vi "Periodic Tasks.vi"(8 "error in":errorcluster) -> ()   [LabVIEW 2020]
doc: "This VI runs in parallel to other tasks. It can contain as many user-defined periodic loops as you need. These can carry out PID or other sorts of timed response."
uses:
  myStates.ctl
  Test VIs/SlipControlStates.ctl
  <vilib>/Rock Robotics/WPI/DriverStation/WPI_DriverStationRobotMode2.ctl
  <vilib>/Rock Robotics/WPI/ThirdParty/REV Robotics/REVLib/Typedef/Spark MAX Control Type.ctl
  4913f956-5bda-4107-8571-b517f3ac16c4.vi
  <vilib>/Rock Robotics/WPI/Utilities/WPI_GetSetVariantRefNum.vi
  <vilib>/Rock Robotics/Network Tables/NT Write Number.vi
  <vilib>/Rock Robotics/Network Tables/NT Read Boolean Array.vi
  <vilib>/Rock Robotics/Network Tables/NT Read Number.vi
  <vilib>/Rock Robotics/Network Tables/NT Read Boolean.vi
  Robot Global Data.vi
  <vilib>/Rock Robotics/Network Tables/NT Write Numeric Array.vi
  <vilib>/Rock Robotics/Network Tables/NT Write String.vi
  <vilib>/Rock Robotics/Network Tables/NT Write Boolean Array.vi
  <vilib>/Comparison/Equal/Equal Functor/Equal Functor.lvclass
panel:
  out "Drivetrain Currents":dbl[](array[numeric])
  out "DEP Right Running Ave":dbl
  out "DEP Left Running Ave":dbl
  out "EXC Right Running Ave":dbl
  out "EXC Left Running Ave":dbl
  # "Click here to set max"
  # "Click here to set min"
  # "Click here to set max"
  # "Click here to set min"
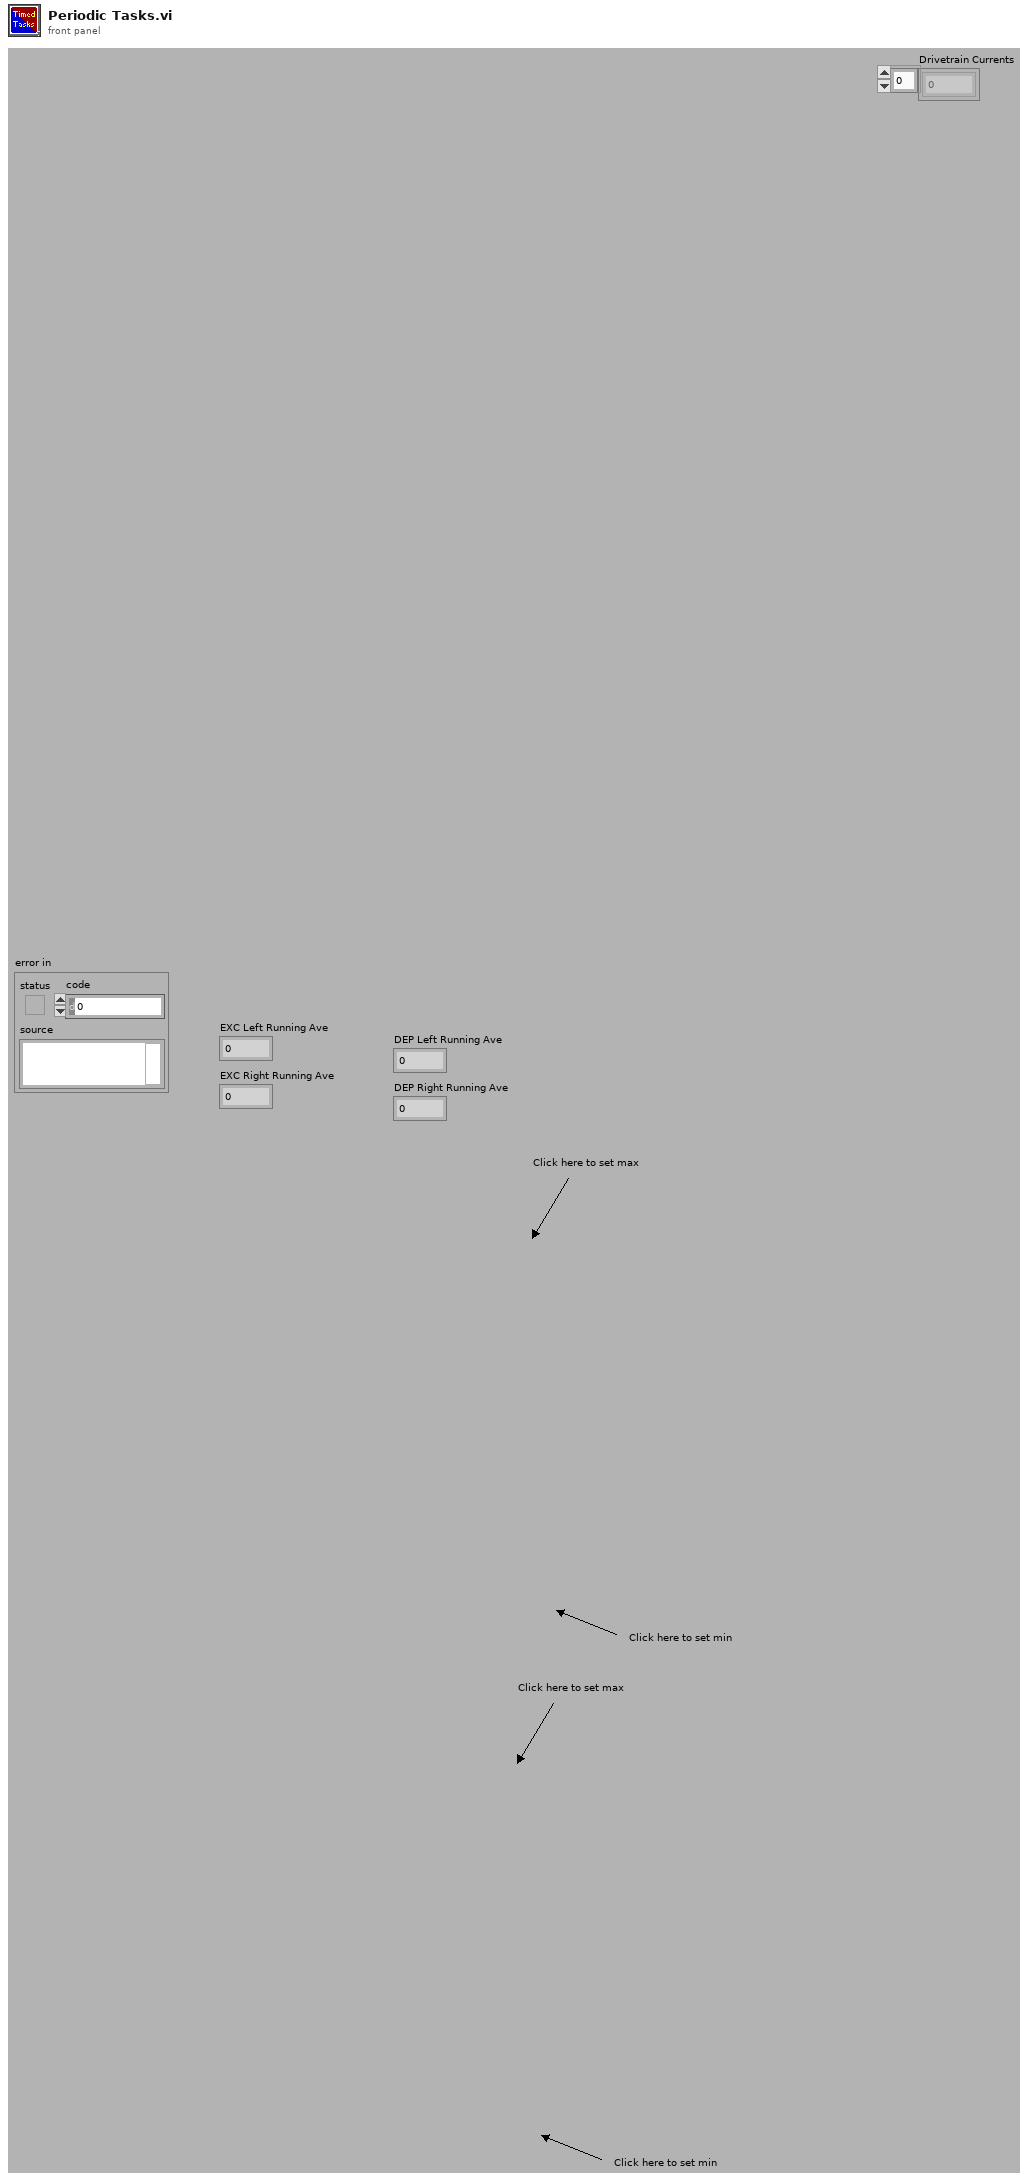
[diagram p1: front panel]
types:
  T1 = typedef "SlipControlStates.ctl" = enum16{"Init", "Grab Time", "Wait", "Grab Time (good)", "Waiting (while run)", "Check", "Grab Time (bad)", "Wait (No Run)"}
  T2 = typedef "myStates.ctl" = enum16{"Init", "Manual Control", "Autonomous Traversal", "Avoid Left", "Avoid Right", "Return to Trench", "EXC Deploy", "EXC Excavate", "EXC Inch", "EXC Index", "EXC Retract", "Drive to Dep", "Approach Berm", "HAD Deploy", "HAD Deposit", "HAD Retract", "Return to EXC"}
  T3 = typedef "WPI_AnalogChannelDevRef.ctl" = cluster{"DevStatus":errorcluster, "Analog Channel":T4}
  T4 = typedef "FPGA_AIChannel.ctl" = enum8{"AI 0", "AI 1", "AI 2", "AI 3", "AI MXP 0", "AI MXP 1", "AI MXP 2", "AI MXP 3", "Invalid"}
  T5 = typedef "WPI_JoystickDevRef.ctl" = cluster{"Device":T6}
  T6 = typedef "WPI_JoystickDeviceEnum.ctl" = enum16{"USB 0", "USB 1", "USB 2", "USB 3", "USB 4", "USB 5"}
  T7 = typedef "Spark MAX Control Type.ctl" = enum16{"Percent VBus", "Voltage", "Velocity", "Position", "Smart Motion", "Current", "Smart Velocity"}
  T8 = typedef "WPI_DriverStationRobotMode2.ctl" = enum16{"Autonomous Disabled", "Autonomous Enabled", "Teleop Disabled", "Teleop Enabled", "Disconnected", "Finish", "Test Disabled", "Test Enabled", "Emergency Stopped"}
  T9 = cluster{"Buttons[0]":bool, "Buttons[1]":bool, "Buttons[2]":bool, "Buttons[3]":bool, "Buttons[4]":bool, "Buttons[5]":bool, "Buttons[6]":bool, "Buttons[7]":bool, "Buttons[8]":bool}
  T10 = cluster{"Axes[0]":dbl, "Axes[1]":dbl, "Axes[2]":dbl, "Axes[3]":dbl, "Axes[4]":dbl, "Axes[5]":dbl, "Axes[6]":dbl, "Axes[7]":dbl, "Axes[8]":dbl}
  T11 = cluster{"Yaw":dbl, "Roll":dbl, "Pitch":dbl, "Heading":dbl, "Fused Heading":dbl}
  T12 = cluster{"Velocity X":dbl, "Velocity Y":dbl, "Velocity Z":dbl, "Displacement X":dbl, "Displacement Y":dbl, "Displacement Z":dbl}
  T13 = typedef "Z900_navX_Flags_HardwareRevTypeDef.ctl" = u8
  T14 = typedef "Z900_navX_Flags_OmnimountConfigTypeDef.ctl" = u8
  T15 = cluster{"Board":cluster{"Who Am I":u8, "Hardware Revision":T13, "Firmware Major Version":u8, "Firmware Minor Version":u8}, "Capability":cluster{"OMNIMOUNT":bool, "YAW_RESET":bool, "VEL_AND_DISP":bool}, "Omnimount Config":T14}
  T16 = cluster{bool[], dbl, dbl, "Left axis value":dbl, "Right axis value":dbl, dbl, "Enum":T1, "current (A)":dbl, "current (A)":dbl, "current (A)":dbl, "current (A)":dbl}
  T17 = cluster{"Want to Drive Out":bool[], "Time Out":dbl, "Front Left Speed Out":dbl, "Back Left Speed Out":dbl, "Front Right Speed Out":dbl, "Back Right Speed Out":dbl, "State Out":T1}
  T18 = typedef "WPI_MotorControlDeviceRef.ctl" = cluster{"DeviceStatus":errorcluster, "Type":T19, "PWM":cluster{"PWM Channel":T20, "DeadBand":T21}, "CAN":cluster{"Device Number":u8, "SetOutput VI Ref":variant, "GetOutput VI Ref":variant, "Enable VI Ref":variant, "Disable VI Ref":variant, "Data":variant}, "Invert":bool, "DIO PWM":cluster{"PWM \"Enable\" Channel":T20, "DIOChannel":T22, "PWM Rate":dbl}}
  T19 = typedef "WPI_MotorControlType.ctl" = enum16{"PWM", "CAN", "DIO PWM"}
  T20 = typedef "FPGA_DIOPWMChannel.ctl" = enum8{"PWM 0", "PWM 1", "PWM 2", "PWM 3", "PWM 4", "PWM 5", "PWM 6", "PWM 7", "PWM 8", "PWM 9", "PWM MXP 0", "PWM MXP 1", "PWM MXP 2", "PWM MXP 3", "PWM MXP 4", "PWM MXP 5", "PWM MXP 6", "PWM MXP 7", "PWM MXP 8", "PWM MXP 9", "Invalid"}
  T21 = typedef "WPI_PWMDeadband.ctl" = cluster{"Name":string, "maxPositivePwm":i32, "minPositivePwm":i32, "centerPwm":i32, "maxNegativePwm":i32, "minNegativePwm":i32, "angularRange":u16}
  T22 = typedef "FPGA_DIOChannel.ctl" = enum8{"DIO 0", "DIO 1", "DIO 2", "DIO 3", "DIO 4", "DIO 5", "DIO 6", "DIO 7", "DIO 8", "DIO 9", "DIO MXP 0", "DIO MXP 1", "DIO MXP 2", "DIO MXP 3", "DIO MXP 4", "DIO MXP 5", "DIO MXP 6", "DIO MXP 7", "DIO MXP 8", "DIO MXP 9", "DIO MXP 10", "DIO MXP 11", "DIO MXP 12", "DIO MXP 13", "DIO MXP 14", "DIO MXP 15", "SPI Port CS1", "SPI Port CS2", "SPI Port CS3", "SPI Port MISO", "SPI Port MOSI", "Invalid"}
  T23 = typedef "WPI_DigitalOutputDevRef.ctl" = cluster{"DIO Channel":T22, "DevStatus":errorcluster}
  T24 = typedef "WPI_RobotDriveDevRef.ctl" = cluster{"DevStatus":errorcluster, "Motors[]":T18[], "Square Inputs":bool, "Max Output":dbl}
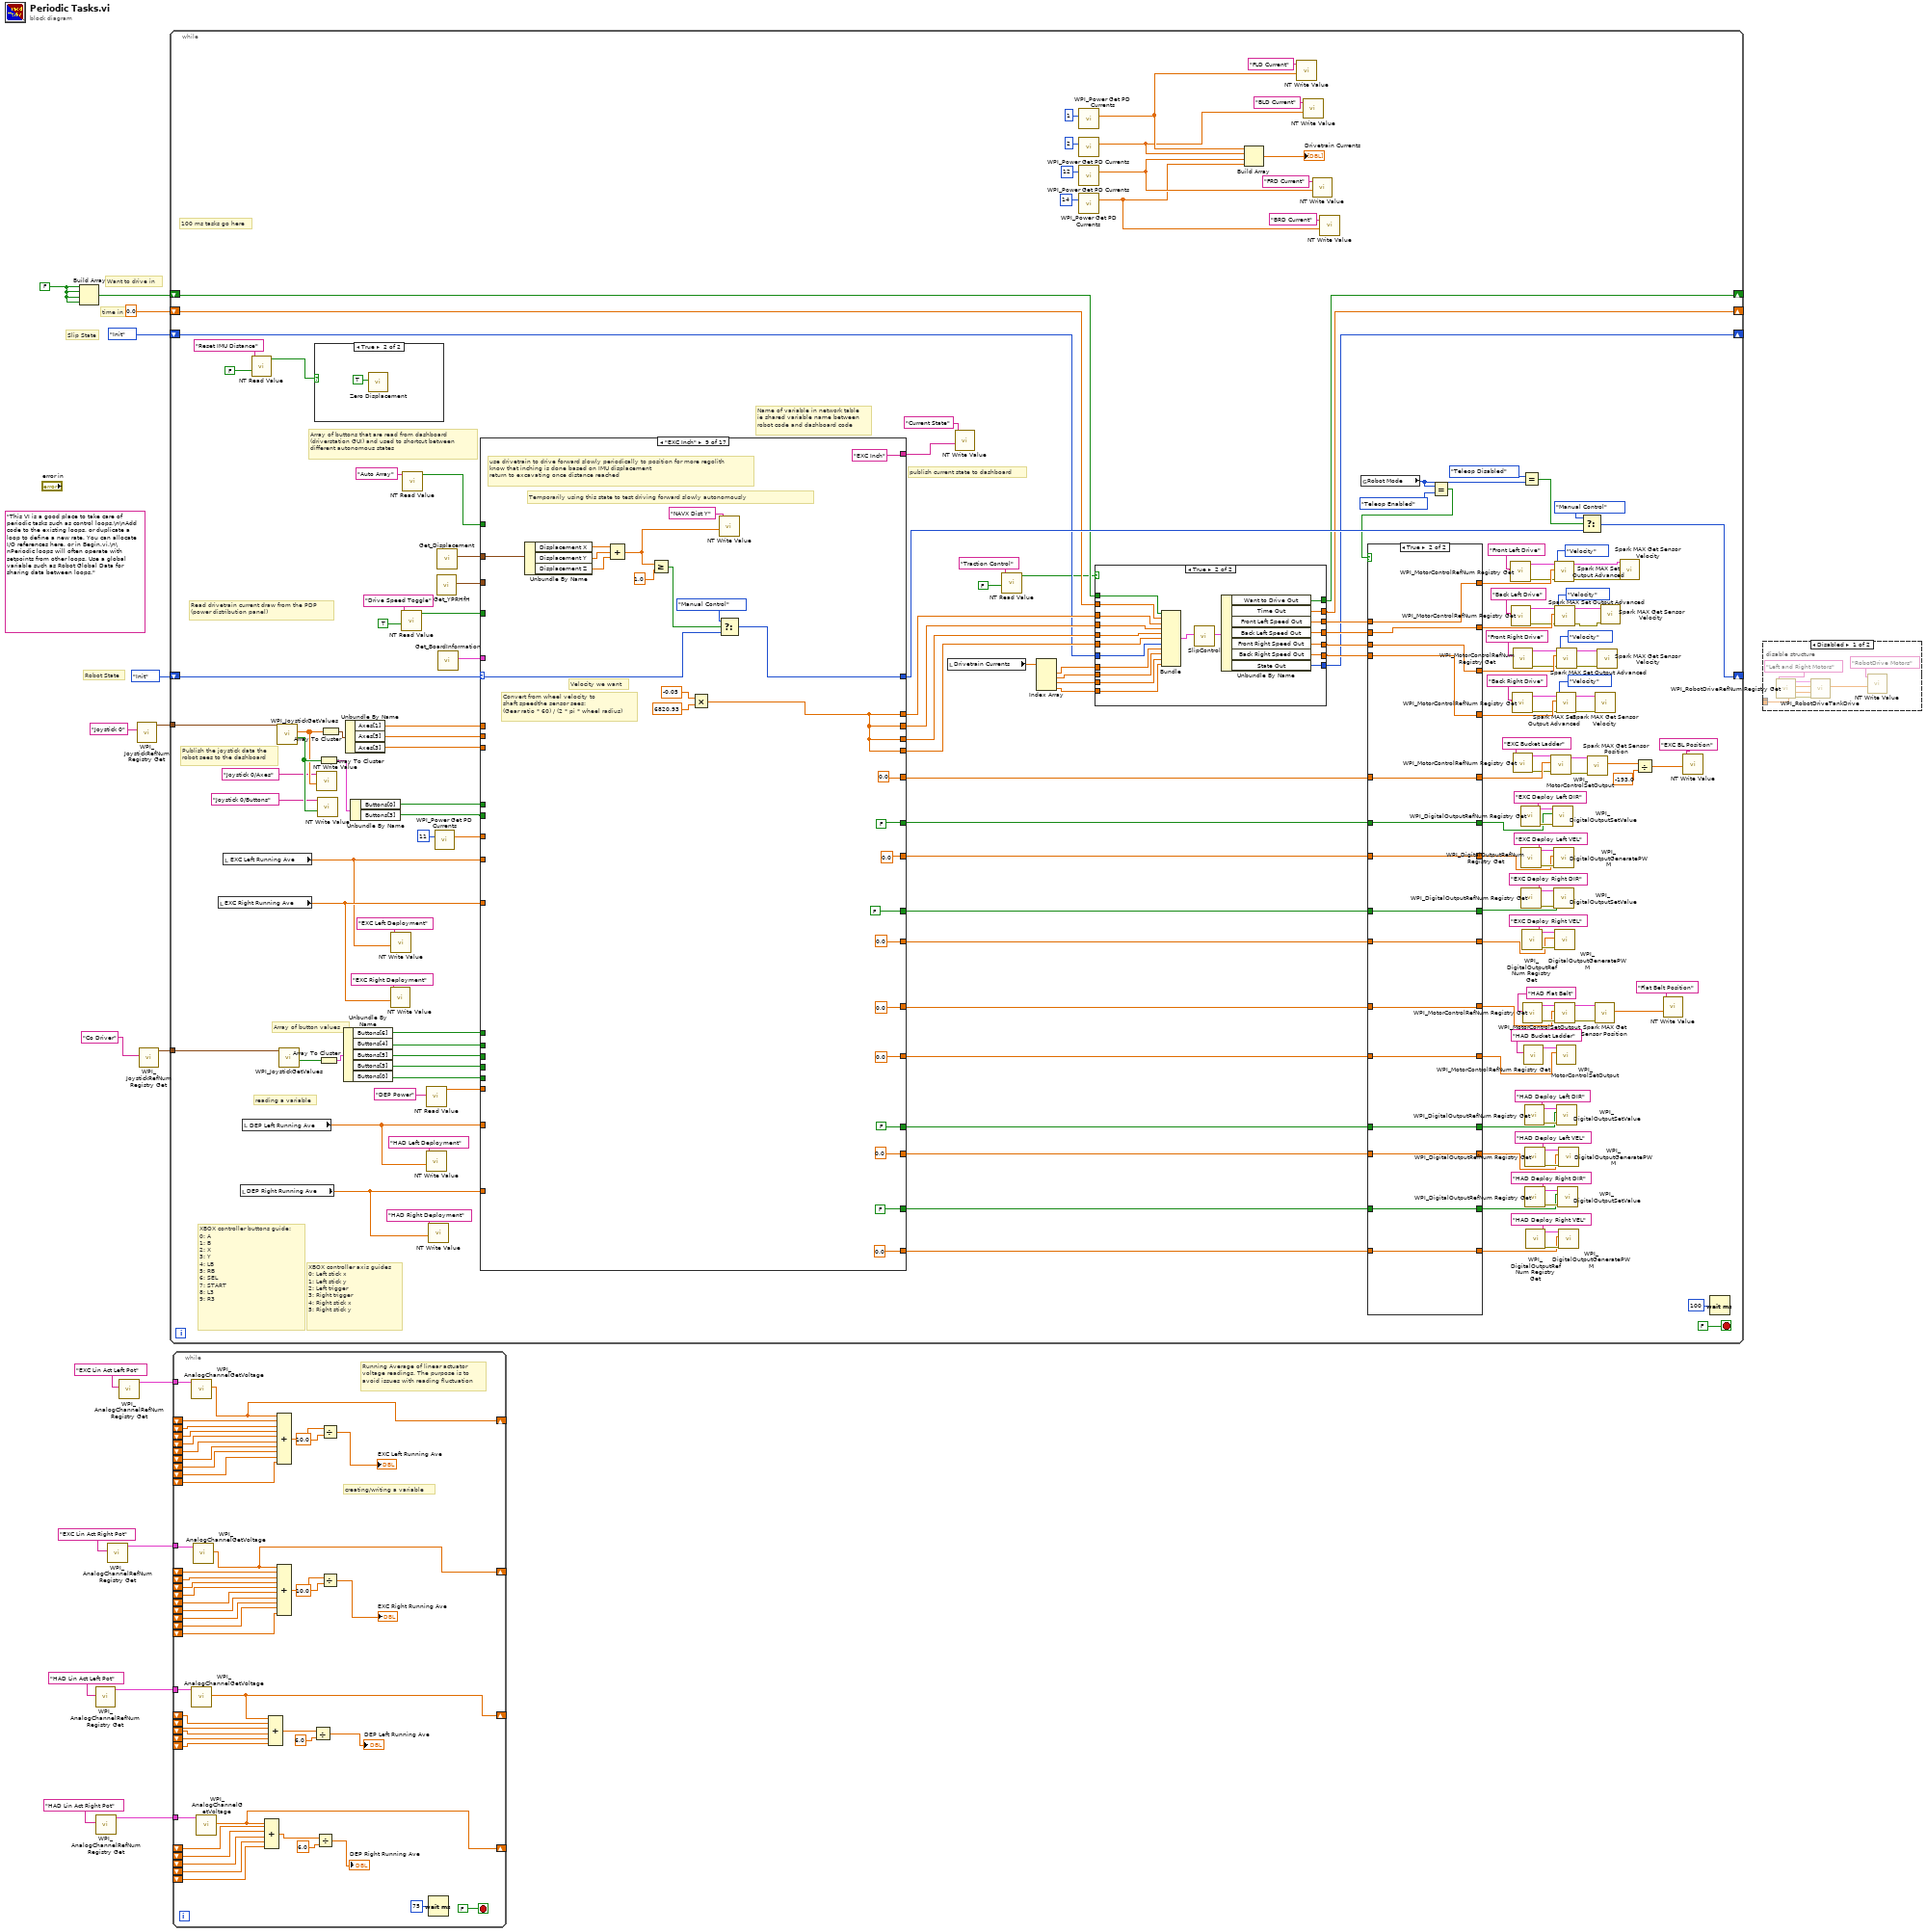
[diagram p0: block diagram]
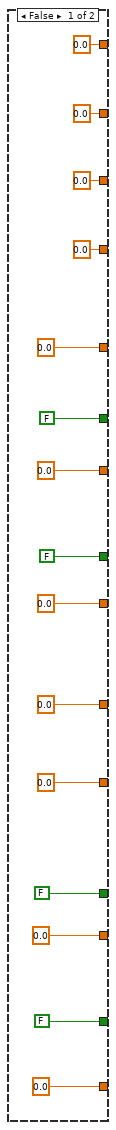
[diagram p5: hidden frame]
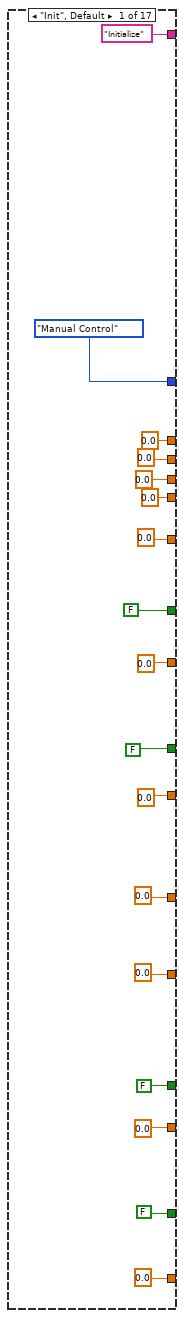
[diagram p6: hidden frame]
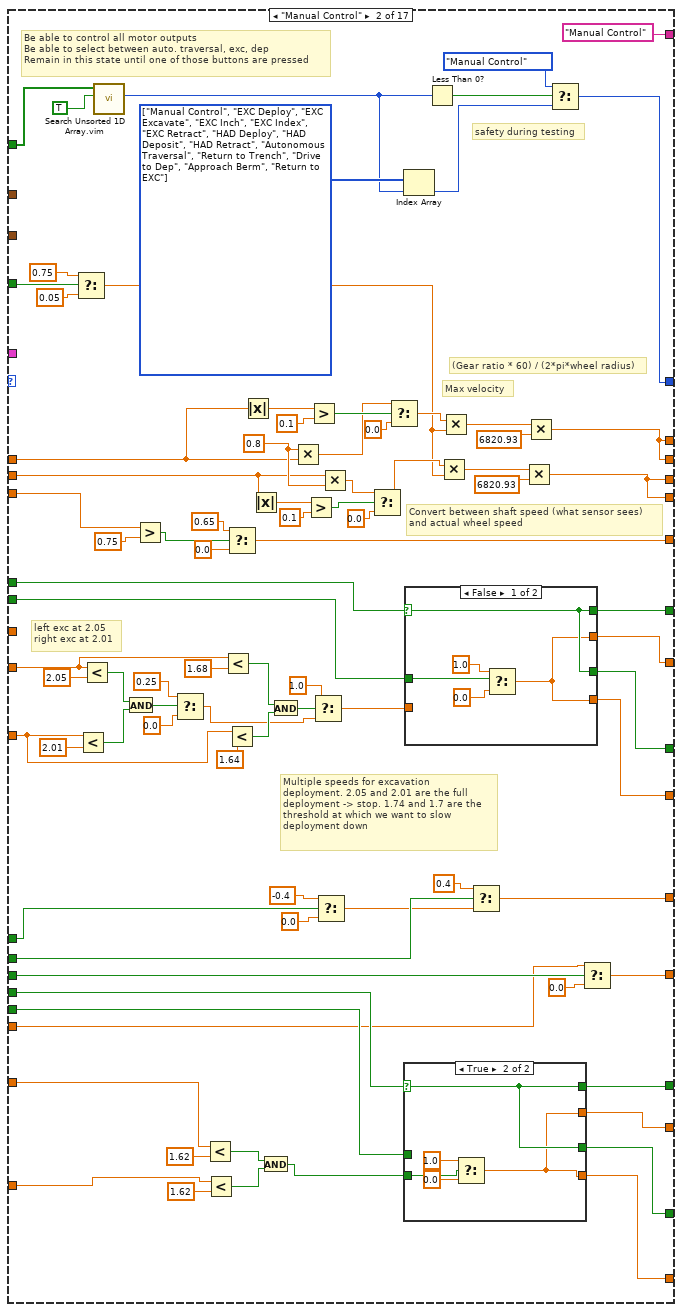
[diagram p7: hidden frame]
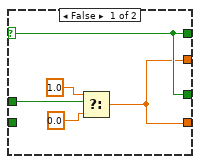
[diagram p8: hidden frame]
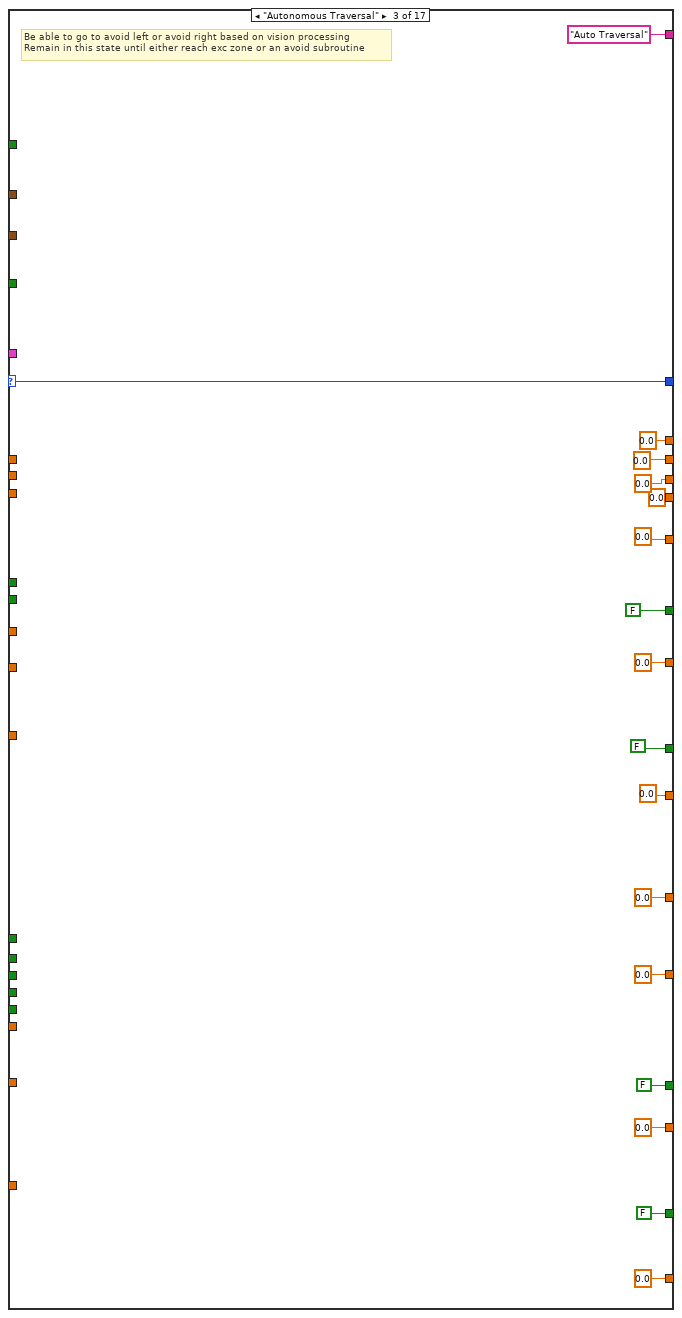
[diagram p10: hidden frame]
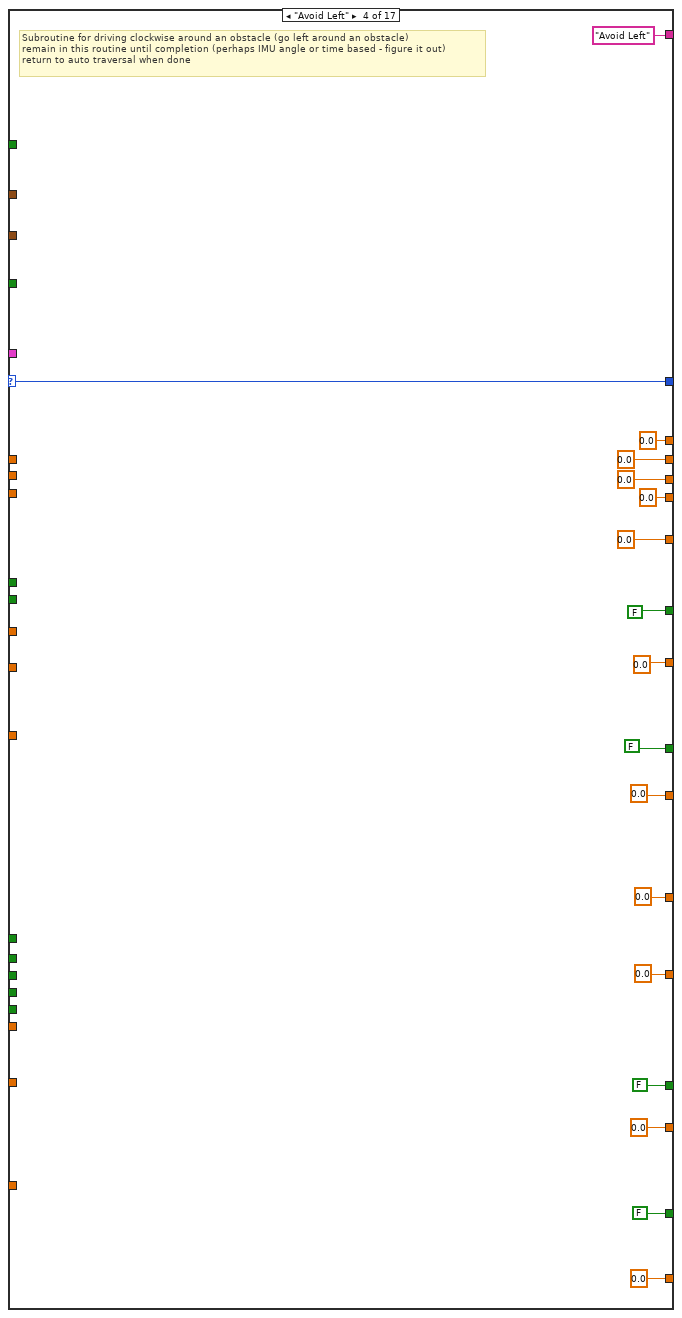
[diagram p11: hidden frame]
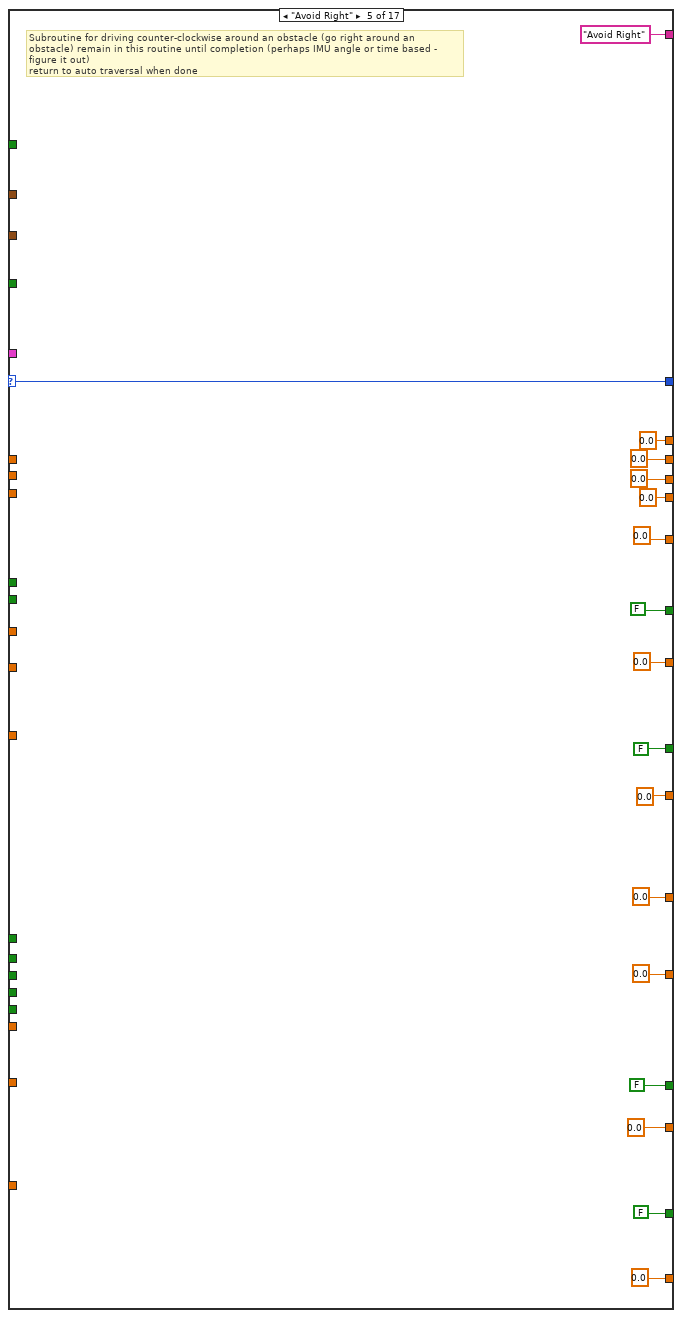
[diagram p12: hidden frame]
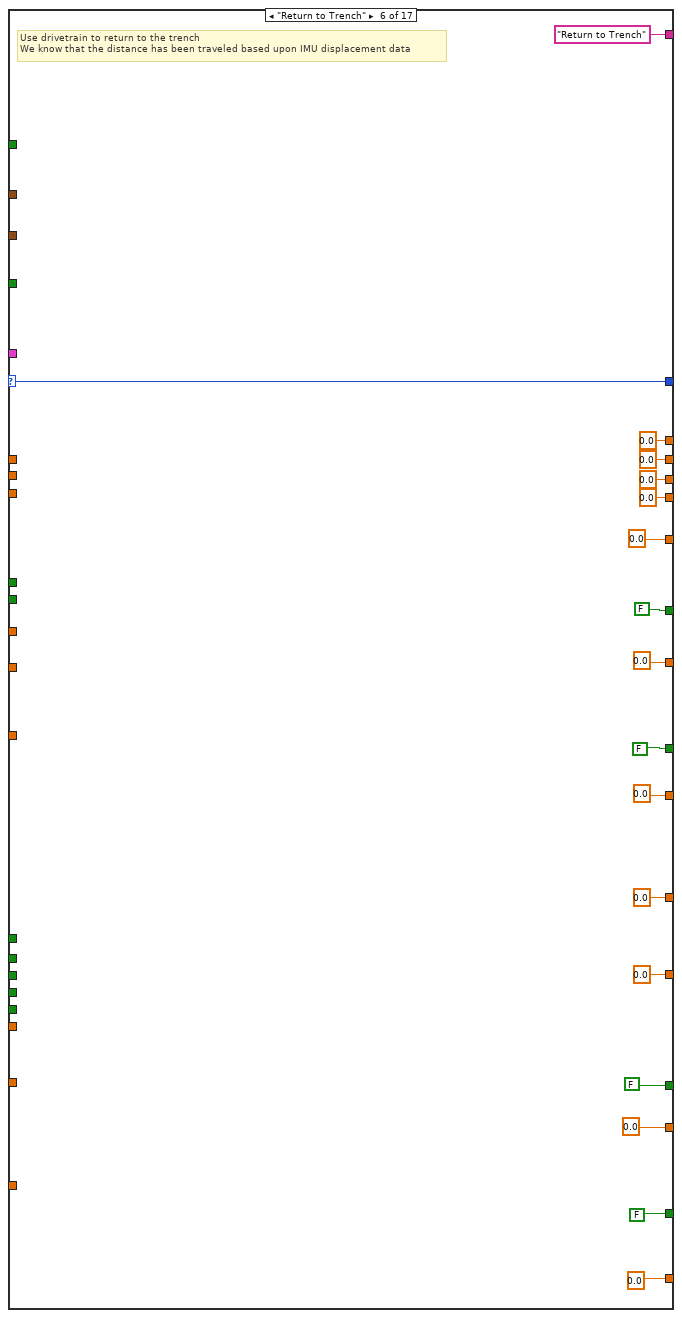
[diagram p13: hidden frame]
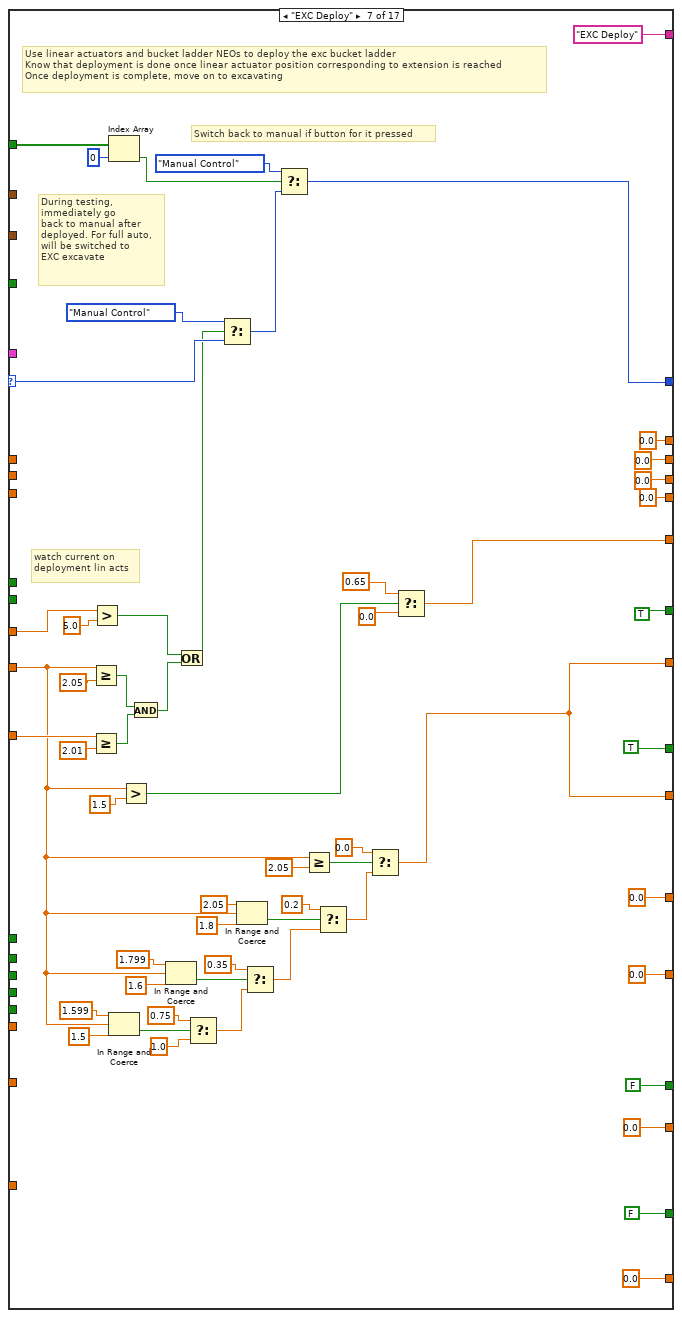
[diagram p14: hidden frame]
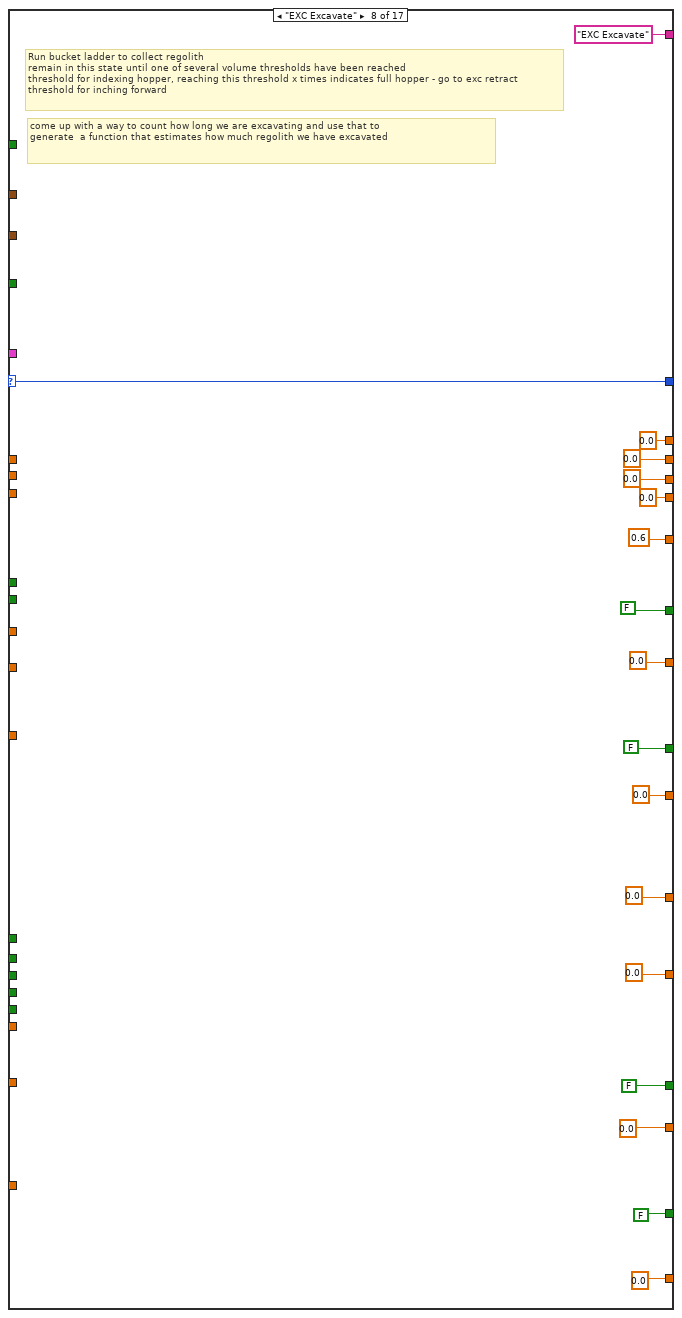
[diagram p15: hidden frame]
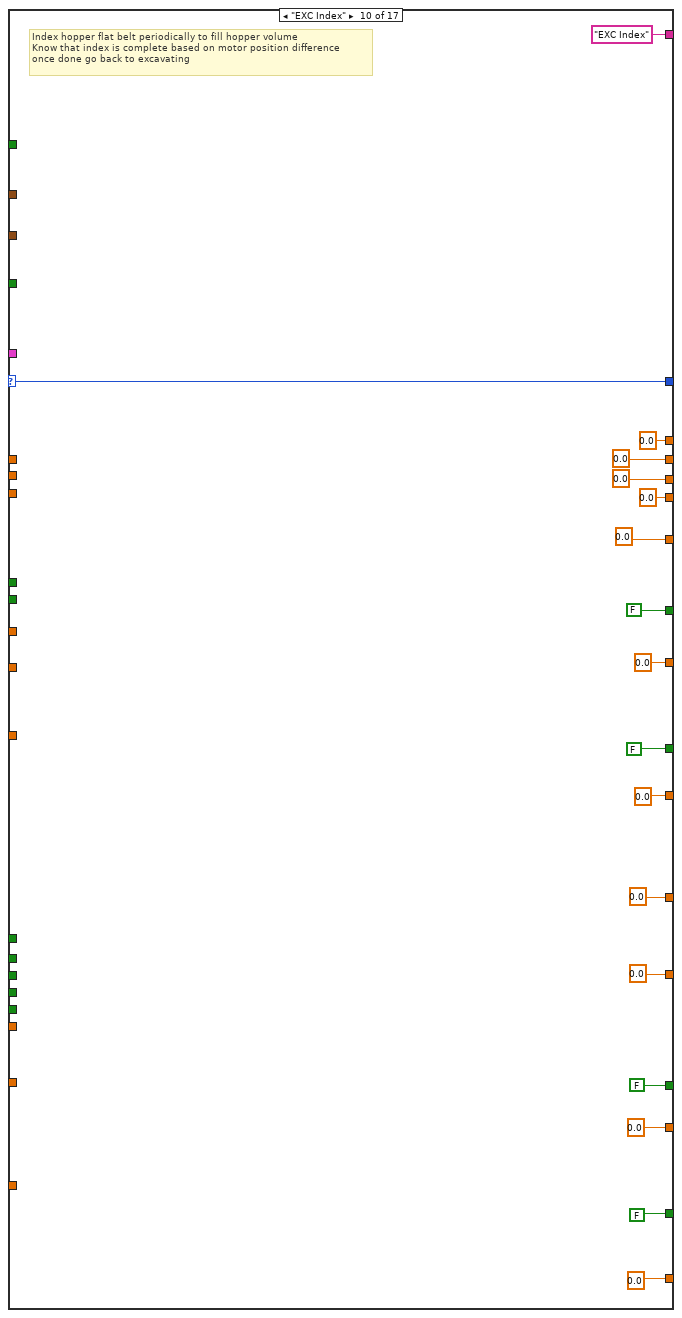
[diagram p16: hidden frame]
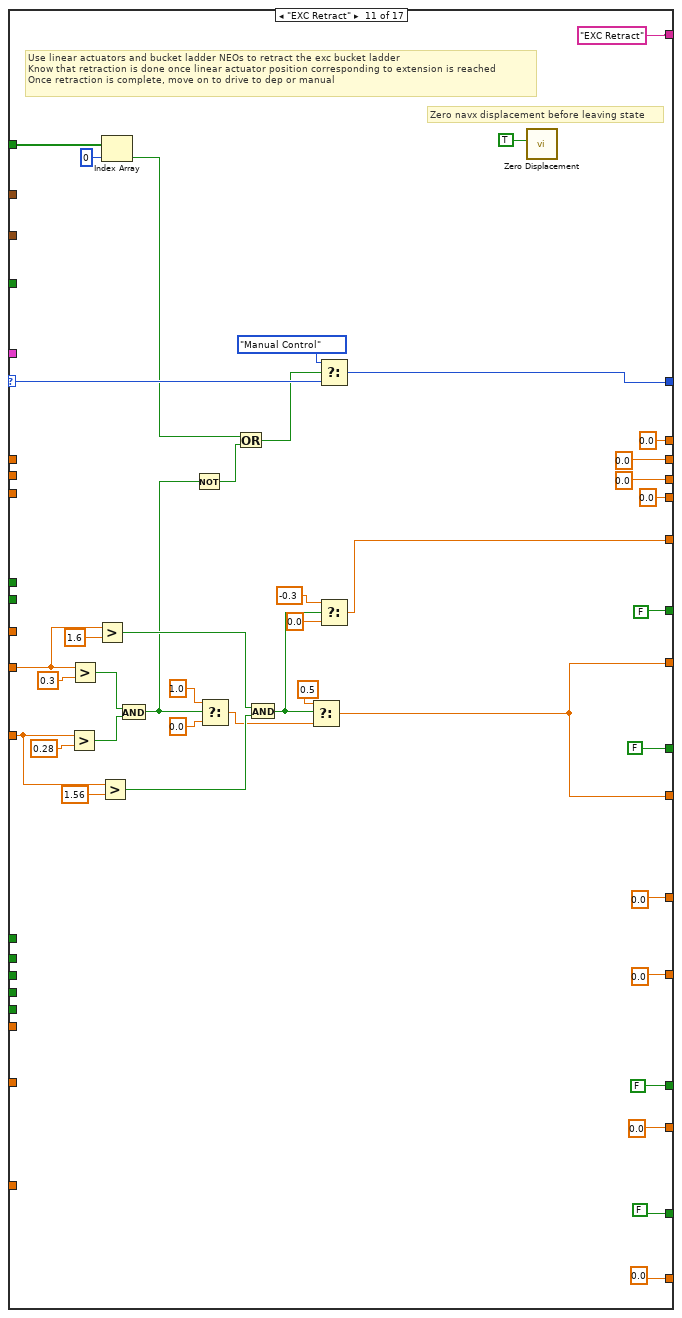
[diagram p17: hidden frame]
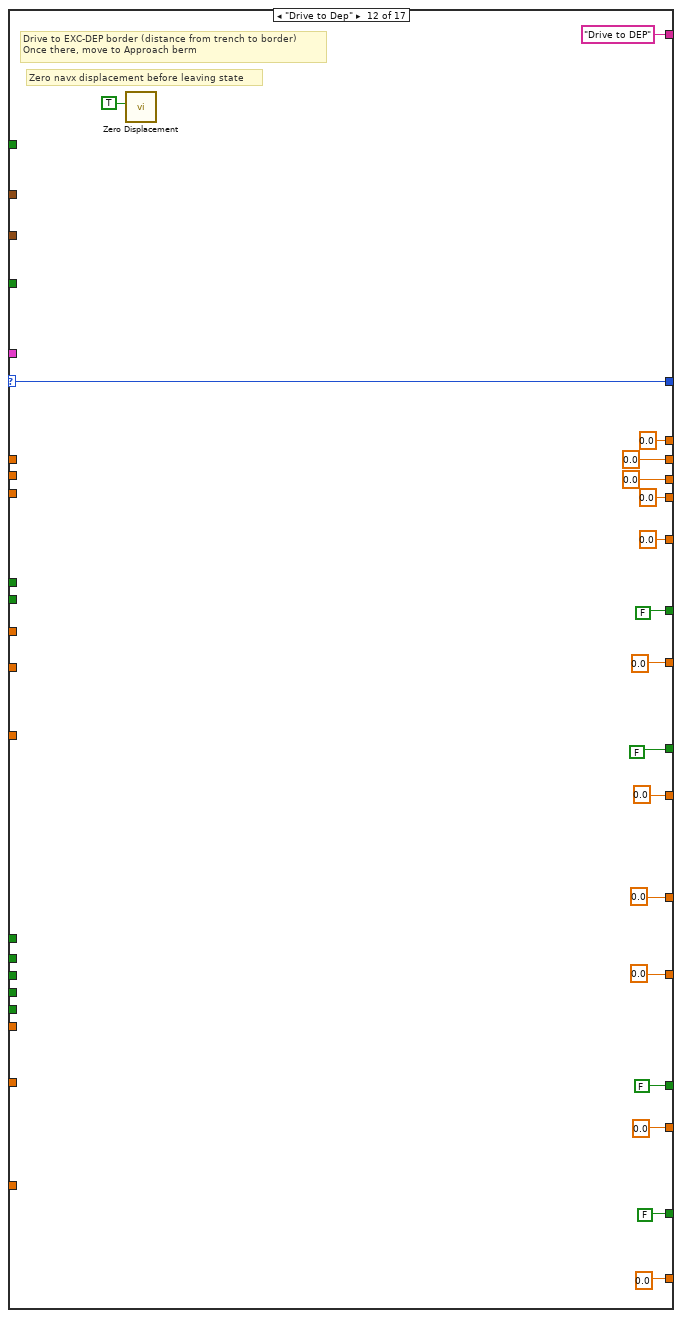
[diagram p18: hidden frame]
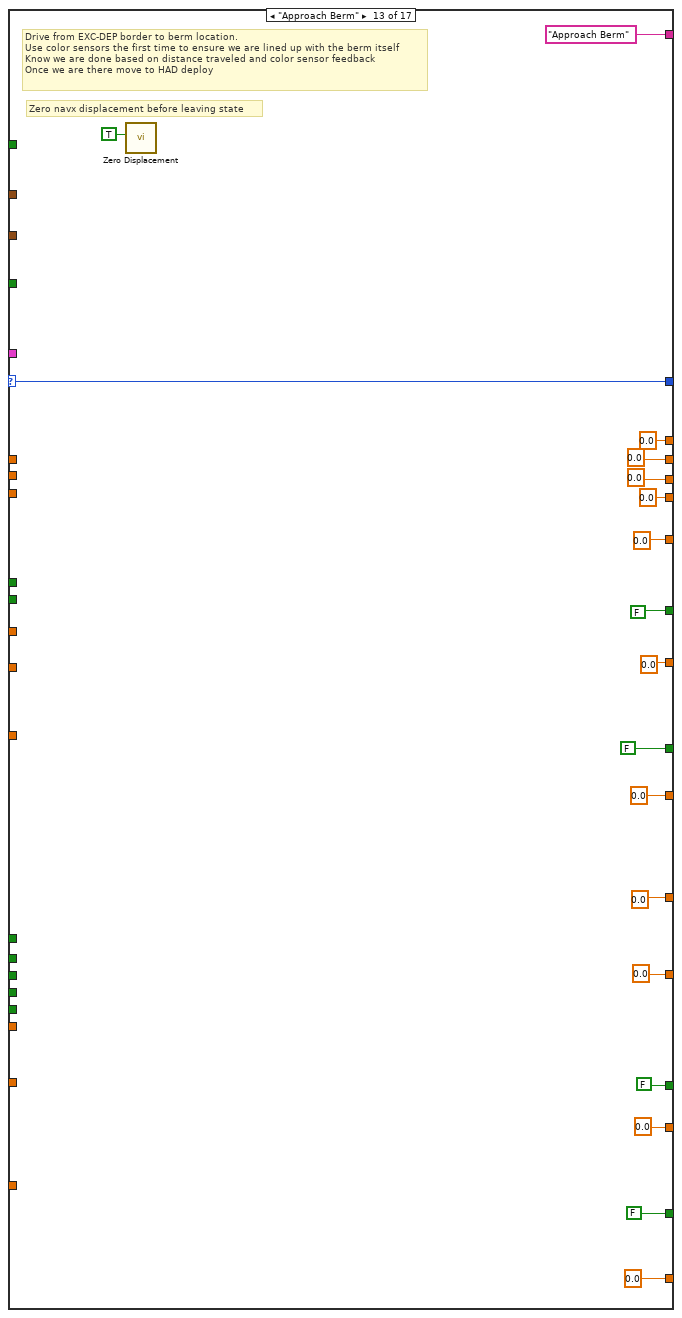
[diagram p19: hidden frame]
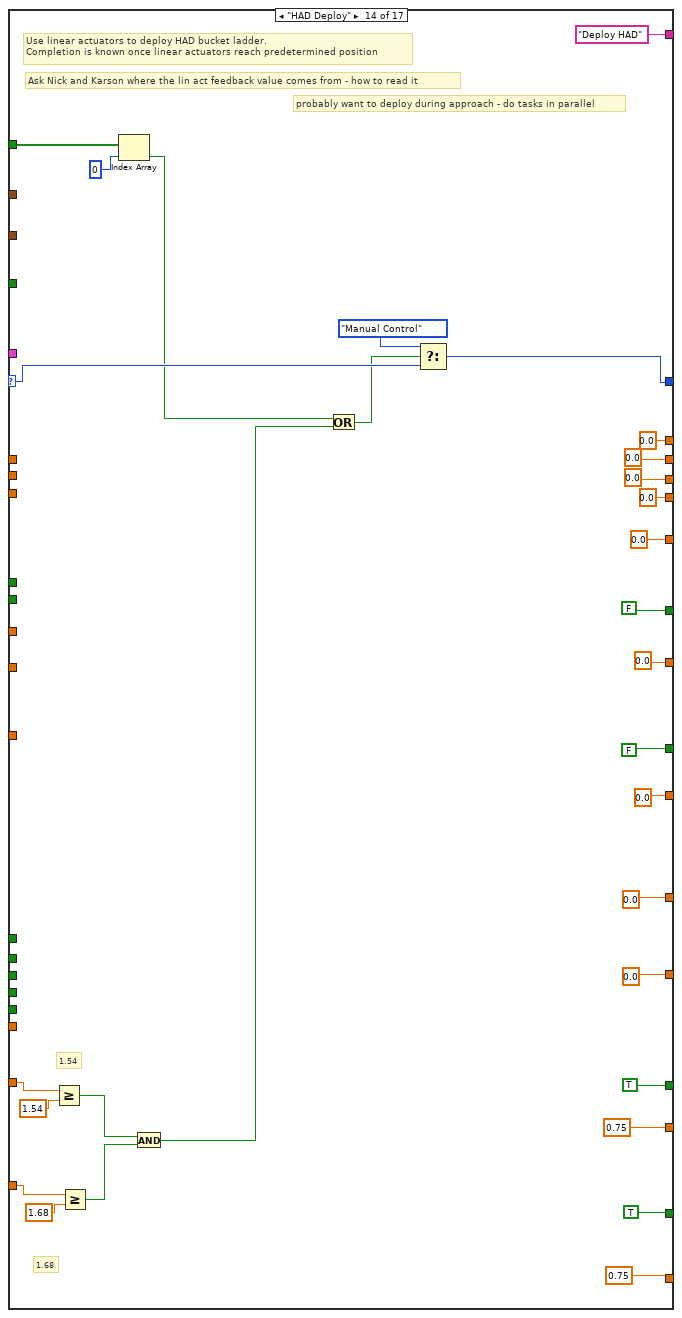
[diagram p20: hidden frame]
diagram:
  w4 = FALSE
  (unwired) "This VI is a good place to take care of periodic tasks such as control loops.\n\nAdd code to the existing loops, or duplicate a loop to define a new rate. You can allocate I/O references here, or in Begin.vi.\n\nPeriodic loops will often operate with setpoints from other loops. Use a global variable such as Robot Global Data for sharing data between loops."
  # "Slip State"
  # "time in"
  # "Want to drive in"
  # "Robot State"
  n1 = Build Array(w4, w4, w4, w4) -> (w3:bool[])
  n2 = call <vilib>:"WPI_AnalogChannelRefNum Registry Get.vi"("refnum name"="HAD Lin Act Left Pot") -> ("AIDeviceRef"=w6:T3)  [unwired: 9 in, 1 out]
  n3 = call <vilib>:"WPI_AnalogChannelRefNum Registry Get.vi"("refnum name"="HAD Lin Act Right Pot") -> ("AIDeviceRef"=w5:T3)  [unwired: 9 in, 1 out]
  n4 = call <vilib>:"WPI_AnalogChannelRefNum Registry Get.vi"("refnum name"="EXC Lin Act Right Pot") -> ("AIDeviceRef"=w7:T3)  [unwired: 9 in, 1 out]
  n5 = call <vilib>:"WPI_AnalogChannelRefNum Registry Get.vi"("refnum name"="EXC Lin Act Left Pot") -> ("AIDeviceRef"=w8:T3)  [unwired: 9 in, 1 out]
  n6 = call <vilib>:"WPI_JoystickRefNum Registry Get.vi"("refnum name"="Joystick 0") -> ("JoystickDevRef"=w15:T5)  [unwired: 1 in, 9 out]
  n7 = call <vilib>:"WPI_JoystickRefNum Registry Get.vi"("refnum name"="Co Driver") -> ("JoystickDevRef"=w13:T5)  [unwired: 1 in, 9 out]
  n8 = while {
    shift-right: [w105] -> _
    shift-left: myStates."Init" -> [w110]
    tunnel: w15 -> [w152]
    tunnel: w13 -> [w151]
    shift-right: [w40] -> _
    shift-left: w3 -> [w59]
    shift-right: [w39] -> _
    shift-left: 0.0 -> [w58]
    shift-right: [w38] -> _
    shift-left: SlipControlStates."Init" ("Enum") -> [w53]
    stop <- FALSE stop-if-true
    # "Read drivetrain current draw from the PDP\n(power distribution panel)"
    # "reading a variable"
    # "Name of variable in network table\nie shared variable name between\nrobot code and dashboard code"
    # "publish current state to dashboard"
    # "XBOX controller axis guides\n0: Left stick x\n1: Left stick y\n2: Left trigger\n3: Right trigger\n4: Right stick x\n5: Right stick y"
    # "XBOX controller buttons guide:\n0: A\n1: B\n2: X\n3: Y\n4: LB\n5: RB\n6: SEL\n7: START\n8: L3\n9: R3"
    # "Array of button values"
    # "Array of buttons that are read from dashboard \n(driverstation GUI) and used to shortcut between \ndifferent autonomous states"
    # "Publish the joystick data the\nrobot sees to the dashboard"
    # "100 ms tasks go here"
    n9 = local read "EXC Right Running Ave"() -> (w114:dbl)
    n10 = local read "EXC Left Running Ave"() -> (w113:dbl)
    n11 = local read "DEP Right Running Ave"() -> (w112:dbl)
    n12 = local read "DEP Left Running Ave"() -> (w111:dbl)
    n13 = call-poly <vilib>:"NT Read Value.vi"("default value"=FALSE, "name"="Reset IMU Distance") -> ("value"=w35:bool)  [unwired: 7 in, 2 out]
    n14 = call <vilib>:"WPI_JoystickGetValues.vi"("JoystickDevRef"=w152) -> ("Buttons"=w167:bool[], "Axes"=w165:dbl[])  [unwired: 6 in, 3 out]
    n15 = call <vilib>:"WPI_JoystickGetValues.vi"("JoystickDevRef"=w151) -> ("Buttons"=w170:bool[])  [unwired: 6 in, 4 out]
    n16 = case shown="True" w35 {
      frame False {
      }
      frame True {
        n17 = call <vilib>:"Zero Displacement.vi"("Zero"=TRUE) -> ()  [unwired: 11 in]
      }
    }
    n18 = call-poly <vilib>:"NT Write Value.vi"("value"=w165, "name"="Joystick 0/Axes" ("Name")) -> ()  [unwired: 9 in, 1 out]
    n19 = call-poly <vilib>:"NT Write Value.vi"("value"=w167, "name"="Joystick 0/Buttons" ("Name")) -> ()  [unwired: 9 in, 1 out]
    n20 = Array To Cluster(array=w167) -> (cluster=w168:T9)
    n21 = Array To Cluster(array=w170) -> (cluster=w169:T9)
    n22 = Array To Cluster(array=w165) -> (cluster=w166:T10)
    n23 = Unbundle By Name(w169) -> ("Buttons[6]"=w120:bool, "Buttons[4]"=w161:bool, "Buttons[5]"=w160:bool, "Buttons[3]"=w159:bool, "Buttons[0]"=w158:bool)
    n24 = Unbundle By Name(w166) -> ("Axes[1]"=w154:dbl, "Axes[5]"=w162:dbl, "Axes[3]"=w155:dbl)
    n25 = Unbundle By Name(w168) -> ("Buttons[0]"=w157:bool, "Buttons[3]"=w156:bool)
    n26 = call-poly <vilib>:"NT Write Value.vi"("value"=w114, "name"="EXC Right Deployment") -> ()  [unwired: 9 in, 1 out]
    n27 = call-poly <vilib>:"NT Write Value.vi"("value"=w113, "name"="EXC Left Deployment") -> ()  [unwired: 9 in, 1 out]
    n28 = call-poly <vilib>:"NT Read Value.vi"("default value"=TRUE, "name"="Drive Speed Toggle") -> ("value"=w61:bool)  [unwired: 7 in, 2 out]
    n29 = call-poly <vilib>:"NT Read Value.vi"("name"="Auto Array") -> ("value"=w125:bool[])  [unwired: 8 in, 2 out]
    n30 = call-poly <vilib>:"NT Read Value.vi"("name"="DEP Power") -> ("value"=w87:dbl)  [unwired: 8 in, 2 out]
    n31 = call-poly <vilib>:"NT Write Value.vi"("value"=w111, "name"="HAD Left Deployment") -> ()  [unwired: 9 in, 1 out]
    n32 = call-poly <vilib>:"NT Write Value.vi"("value"=w112, "name"="HAD Right Deployment") -> ()  [unwired: 9 in, 1 out]
    n33 = call <vilib>:"WPI_Power Get PD Currents.vi"("PD Channel"=11) -> ("current (A)"=w115:dbl)  [unwired: 11 in, 3 out]
    n34 = call <vilib>:"Get_YPRHfH.vi"() -> ("YRPHfH"=w33:T11)  [unwired: 11 in]
    n35 = call <vilib>:"Get_Displacement.vi"() -> ("Displacement"=w34:T12)  [unwired: 11 in]
    n36 = call <vilib>:"Get_BoardInformation.vi"() -> ("Board Information"=w32:T15)  [unwired: 11 in]
    n37 = case shown="\"EXC Inch\"" w110 {
      selector: w110 -> [_ _ w383 w400 w417 w436 w457 w508 w529 w551 w573 w610 w628 w650 w676 w694 w723]
      tunnel: [myStates."Manual Control" w338 w383 w400 w417 w436 w490 w508 w528 w551 w572 w610 w628 w649 w676 w693 w723] -> w106
      tunnel: [0.0 ("Output") w329 0.0 ("Output") 0.0 ("Output") 0.0 ("Output") 0.0 ("Output") w455 0.6 ("Output") 0.0 ("Output") 0.0 ("Output") w577 0.0 ("Output") 0.0 ("Output") 0.0 ("Output") 0.0 ("Output") 0.0 ("Output") 0.0 ("Output")] -> w149
      tunnel: [0.0 ("Left axis value") w278 0.0 ("Left axis value") 0.0 ("Left axis value") 0.0 ("Left axis value") 0.0 ("Left axis value") 0.0 ("Left axis value") 0.0 ("Left axis value") w533 0.0 ("Left axis value") 0.0 ("Left axis value") 0.0 ("Left axis value") 0.0 ("Left axis value") 0.0 ("Left axis value") 0.0 ("Left axis value") 0.0 ("Left axis value") 0.0 ("Left axis value")] -> w56
      tunnel: [0.0 ("Right axis value") w277 0.0 ("Right axis value") 0.0 ("Right axis value") 0.0 ("Right axis value") 0.0 ("Right axis value") 0.0 ("Right axis value") 0.0 ("Right axis value") w533 0.0 ("Right axis value") 0.0 ("Right axis value") 0.0 ("Right axis value") 0.0 ("Right axis value") 0.0 ("Right axis value") 0.0 ("Right axis value") 0.0 ("Right axis value") 0.0 ("Right axis value")] -> w55
      tunnel: w154 -> [_ w301 _ _ _ _ _ _ _ _ _ _ _ _ _ _ _]
      tunnel: w162 -> [_ w296 _ _ _ _ _ _ _ _ _ _ _ _ _ _ _]
      tunnel: w155 -> [_ w361 _ _ _ _ _ _ _ _ _ _ _ _ _ _ _]
      tunnel: w157 -> [_ w354 _ _ _ _ _ _ _ _ _ _ _ _ _ _ _]
      tunnel: w156 -> [_ w353 _ _ _ _ _ _ _ _ _ _ _ _ _ _ _]
      tunnel: w161 -> [_ w358 _ _ _ _ _ _ _ _ _ _ _ _ _ _ _]
      tunnel: [FALSE ("Buttons[0]") w352 FALSE ("Buttons[0]") FALSE ("Buttons[0]") FALSE ("Buttons[0]") FALSE ("Buttons[0]") TRUE ("Buttons[0]") FALSE ("Buttons[0]") FALSE ("Buttons[0]") FALSE ("Buttons[0]") FALSE ("Buttons[0]") FALSE ("Buttons[0]") FALSE ("Buttons[0]") FALSE ("Buttons[0]") FALSE ("Buttons[0]") FALSE ("Buttons[0]") FALSE ("Buttons[0]")] -> w148
      tunnel: w160 -> [_ w357 _ _ _ _ _ _ _ _ _ _ _ _ _ _ _]
      tunnel: [FALSE ("Buttons[1]") w349 FALSE ("Buttons[1]") FALSE ("Buttons[1]") FALSE ("Buttons[1]") FALSE ("Buttons[1]") TRUE ("Buttons[1]") FALSE ("Buttons[1]") FALSE ("Buttons[1]") FALSE ("Buttons[1]") FALSE ("Buttons[1]") FALSE ("Buttons[1]") FALSE ("Buttons[1]") FALSE ("Buttons[1]") FALSE ("Buttons[1]") FALSE ("Buttons[1]") FALSE ("Buttons[1]")] -> w146
      tunnel: [0.0 ("f") w350 0.0 ("f") 0.0 ("f") 0.0 ("f") 0.0 ("f") w462 0.0 ("f") 0.0 ("f") 0.0 ("f") w581 0.0 ("f") 0.0 ("f") 0.0 ("f") 0.0 ("f") 0.0 ("f") 0.0 ("f")] -> w145
      tunnel: [0.0 ("f") w351 0.0 ("f") 0.0 ("f") 0.0 ("f") 0.0 ("f") w462 0.0 ("f") 0.0 ("f") 0.0 ("f") w581 0.0 ("f") 0.0 ("f") 0.0 ("f") 0.0 ("f") 0.0 ("f") 0.0 ("f")] -> w147
      tunnel: [FALSE ("Value") w346 FALSE ("Value") FALSE ("Value") FALSE ("Value") FALSE ("Value") FALSE ("Value") FALSE ("Value") FALSE ("Value") FALSE ("Value") FALSE ("Value") FALSE ("Value") FALSE ("Value") TRUE ("Value") FALSE ("Value") FALSE ("Value") FALSE ("Value")] -> w142
      tunnel: [sgl 0.0 ("PWM Duty Cycle") w344 sgl 0.0 ("PWM Duty Cycle") sgl 0.0 ("PWM Duty Cycle") sgl 0.0 ("PWM Duty Cycle") sgl 0.0 ("PWM Duty Cycle") sgl 0.0 ("PWM Duty Cycle") sgl 0.0 ("PWM Duty Cycle") sgl 0.0 ("PWM Duty Cycle") sgl 0.0 ("PWM Duty Cycle") sgl 0.0 ("PWM Duty Cycle") sgl 0.0 ("PWM Duty Cycle") sgl 0.0 ("PWM Duty Cycle") sgl 0.75 ("PWM Duty Cycle") sgl 0.0 ("PWM Duty Cycle") sgl 0.75 ("PWM Duty Cycle") sgl 0.0 ("PWM Duty Cycle")] -> w141
      tunnel: [FALSE ("Value") w345 FALSE ("Value") FALSE ("Value") FALSE ("Value") FALSE ("Value") FALSE ("Value") FALSE ("Value") FALSE ("Value") FALSE ("Value") FALSE ("Value") FALSE ("Value") FALSE ("Value") TRUE ("Value") FALSE ("Value") FALSE ("Value") FALSE ("Value")] -> w140
      tunnel: [sgl 0.0 ("PWM Duty Cycle") w343 sgl 0.0 ("PWM Duty Cycle") sgl 0.0 ("PWM Duty Cycle") sgl 0.0 ("PWM Duty Cycle") sgl 0.0 ("PWM Duty Cycle") sgl 0.0 ("PWM Duty Cycle") sgl 0.0 ("PWM Duty Cycle") sgl 0.0 ("PWM Duty Cycle") sgl 0.0 ("PWM Duty Cycle") sgl 0.0 ("PWM Duty Cycle") sgl 0.0 ("PWM Duty Cycle") sgl 0.0 ("PWM Duty Cycle") sgl 0.75 ("PWM Duty Cycle") sgl 0.0 ("PWM Duty Cycle") sgl 0.75 ("PWM Duty Cycle") sgl 0.0 ("PWM Duty Cycle")] -> w139
      tunnel: [0.0 ("f") w356 0.0 ("f") 0.0 ("f") 0.0 ("f") 0.0 ("f") 0.0 ("f") 0.0 ("f") 0.0 ("f") 0.0 ("f") 0.0 ("f") 0.0 ("f") 0.0 ("f") 0.0 ("f") 0.0 ("f") 0.0 ("f") 0.0 ("f")] -> w144
      tunnel: [0.0 ("f") w355 0.0 ("f") 0.0 ("f") 0.0 ("f") 0.0 ("f") 0.0 ("f") 0.0 ("f") 0.0 ("f") 0.0 ("f") 0.0 ("f") 0.0 ("f") 0.0 ("f") 0.0 ("f") 0.0 ("f") 0.0 ("f") 0.0 ("f")] -> w143
      tunnel: w159 -> [_ w348 _ _ _ _ _ _ _ _ _ _ _ _ _ _ _]
      tunnel: w158 -> [_ w347 _ _ _ _ _ _ _ _ _ _ _ _ _ _ _]
      tunnel: w113 -> [_ w321 _ _ _ _ w456 _ _ _ w589 _ _ _ _ _ _]
      tunnel: w114 -> [_ w319 _ _ _ _ w464 _ _ _ w587 _ _ _ _ _ _]
      tunnel: w125 -> [_ w311 _ _ _ _ w494 _ _ _ w576 _ _ w651 _ w706 _]
      tunnel: w120 -> [_ w309 _ _ _ _ _ _ _ _ _ _ _ _ _ _ _]
      tunnel: w115 -> [_ _ _ _ _ _ w460 _ _ _ _ _ _ _ _ _ _]
      tunnel: w112 -> [_ w303 _ _ _ _ _ _ _ _ _ _ _ w656 _ w700 _]
      tunnel: w111 -> [_ w304 _ _ _ _ _ _ _ _ _ _ _ w659 _ w703 _]
      tunnel: ["Initialize" ("Current State") "Manual Control" ("Current State") "Auto Traversal" ("Current State") "Avoid Left" ("Current State") "Avoid Right" ("Current State") "Return to Trench" ("Current State") "EXC Deploy" ("Current State") "EXC Excavate" ("Current State") "EXC Inch" ("Current State") "EXC Index" ("Current State") "EXC Retract" ("Current State") "Drive to DEP" ("Current State") "Approach Berm" ("Current State") "Deploy HAD" ("Current State") "HAD Deposit" ("Current State") "HAD Retract" ("Current State") "Return to EXC" ("Current State")] -> w89
      tunnel: [0.0 w278 0.0 0.0 0.0 0.0 0.0 0.0 w533 0.0 0.0 0.0 0.0 0.0 0.0 0.0 0.0] -> w57
      tunnel: [0.0 w277 0.0 0.0 0.0 0.0 0.0 0.0 w533 0.0 0.0 0.0 0.0 0.0 0.0 0.0 0.0] -> w54
      tunnel: w87 -> [_ w289 _ _ _ _ _ _ _ _ _ _ _ _ _ _ _]
      tunnel: w61 -> [_ w281 _ _ _ _ _ _ _ _ _ _ _ _ _ _ _]
      tunnel: w34 -> [_ _ _ _ _ _ _ _ w526 _ _ _ _ _ _ _ _]
      tunnel: w33 -> [_ _ _ _ _ _ _ _ _ _ _ _ _ _ _ _ _]
      tunnel: w32 -> [_ _ _ _ _ _ _ _ _ _ _ _ _ _ _ _ _]
      frame "Init", Default {
      }
      frame "Manual Control" {
        w341 = T2[] [enum."Manual Control", enum."EXC Deploy", enum."EXC Excavate", enum."EXC Inch", enum."EXC Index", enum."EXC Retract", enum."HAD Deploy", enum."HAD Deposit", enum."HAD Retract", enum."Autonomous Traversal", enum."Return to Trench", enum."Drive to Dep", enum."Approach Berm", enum."Return to EXC"] items=["Init", "Manual Control", "Autonomous Traversal", "Avoid Left", "Avoid Right", "Return to Trench", "EXC Deploy", "EXC Excavate", "EXC Inch", "EXC Index", "EXC Retract", "Drive to Dep", "Approach Berm", "HAD Deploy", "HAD Deposit", "HAD Retract", "Return to EXC"]
        w362 = 0.8 ("x")
        # "(Gear ratio * 60) / (2*pi*wheel radius)"
        # "Max velocity"
        # "Convert between shaft speed (what sensor sees)\nand actual wheel speed"
        # "left exc at 2.05\nright exc at 2.01"
        # "Multiple speeds for excavation\ndeployment. 2.05 and 2.01 are the full\ndeployment -> stop. 1.74 and 1.7 are the\nthreshold at which we want to slow \ndeployment down"
        # "safety during testing"
        # "Be able to control all motor outputs\nBe able to select between auto. traversal, exc, dep\nRemain in this state until one of those buttons are pressed"
        n38 = Select(t=0.75, s=w281, f=0.05) -> (s? t:f=w276:dbl)
        n39 = Less?(x=w319, y=2.01) -> (x < y?=w325:bool)
        n40 = Less?(x=w321, y=2.05) -> (x < y?=w326:bool)
        n41 = call "Search Unsorted 1D Array.vim"("element"=TRUE, "unsorted 1D array"=w311) -> ("index of element"=w340:i32)  [unwired: 9 in]
        n42 = And(x=w326, y=w325) -> (x .and. y?=w324:bool)
        n43 = Greater?(x=w361, y=0.75) -> (0:w331:bool)
        n44 = Select(t=0.25, s=w324, f=0.0) -> (s? t:f=w313:dbl)
        n45 = Less?(x=w304, y=1.62) -> (x < y?=w334:bool)
        n46 = Less?(x=w303, y=1.62) -> (x < y?=w335:bool)
        n47 = Less?(x=w321, y=1.68) -> (x < y?=w316:bool)
        n48 = Select(t=0.65 ("value"), s=w331, f=0.0) -> (s? t:f=w329:dbl)
        n49 = Less?(x=w319, y=1.64) -> (x < y?=w315:bool)
        n50 = Absolute Value(x=w301) -> (abs(x)=w290:dbl)
        n51 = Absolute Value(x=w296) -> (abs(x)=w291:dbl)
        n52 = And(x=w334, y=w335) -> (x .and. y?=w333:bool)
        n53 = And(x=w316, y=w315) -> (x .and. y?=w317:bool)
        n54 = Multiply(x=w362, y=w301) -> (x*y=w298:dbl)
        n55 = Greater?(x=w291, y=0.1) -> (0:w292:bool)
        n56 = Greater?(x=w290, y=0.1) -> (0:w299:bool)
        n57 = Select(t=1.0, s=w317, f=w313) -> (s? t:f=w312:dbl)
        n58 = Select(t=-0.4, s=w309, f=0.0) -> (s? t:f=w306:dbl)
        n59 = Multiply(x=w296, y=w362) -> (x*y=w293:dbl)
        n60 = Select(t=w293, s=w292, f=0.0) -> (s? t:f=w283:dbl)
        n61 = Select(t=w298, s=w299, f=0.0) -> (s? t:f=w284:dbl)
        n62 = Index Array(array=w341, index=w340) -> (element=w339:T2)
        n63 = case shown="True" w348 {
          selector: w348 -> [w367 w372]
          tunnel: w347 -> [w366 _]
          tunnel: [w367 w372] -> w346
          tunnel: [w363 w368] -> w344
          tunnel: [w363 w368] -> w343
          tunnel: [w367 w372] -> w345
          tunnel: w333 -> [_ w371]
          frame False {
            n64 = Select(t=1.0, s=w366, f=0.0) -> (s? t:f=w363:dbl)
          }
          frame True {
            n65 = Select(t=1.0, s=w371, f=0.0) -> (s? t:f=w368:dbl)
          }
        }
        n66 = case shown="False" w354 {
          selector: w354 -> [w377 w379]
          tunnel: w353 -> [w376 _]
          tunnel: [w377 w379] -> w352
          tunnel: [w373 w378] -> w351
          tunnel: [w373 w378] -> w350
          tunnel: [w377 w379] -> w349
          tunnel: w312 -> [_ w378]
          frame False {
            n67 = Select(t=1.0, s=w376, f=0.0) -> (s? t:f=w373:dbl)
          }
          frame True {
          }
        }
        n68 = Less Than 0?(x=w340) -> (x < 0?=w305:bool)
        n69 = Multiply(x=w283, y=w276) -> (x*y=w285:dbl)
        n70 = Multiply(x=w284, y=w276) -> (x*y=w288:dbl)
        n71 = Select(t=0.4, s=w358, f=w306) -> (s? t:f=w356:dbl)
        n72 = Multiply(x=w285, y=6820.93) -> (x*y=w277:dbl)
        n73 = Multiply(x=w288, y=6820.93) -> (x*y=w278:dbl)
        n74 = Select(t=myStates."Manual Control", s=w305, f=w339) -> (s? t:f=w338:T2)
        n75 = Select(t=w289, s=w357, f=0.0) -> (s? t:f=w355:dbl)
      }
      frame "Autonomous Traversal" {
        # "Be able to go to avoid left or avoid right based on vision processing\nRemain in this state until either reach exc zone or an avoid subroutine"
      }
      frame "Avoid Left" {
        # "Subroutine for driving clockwise around an obstacle (go left around an obstacle)\nremain in this routine until completion (perhaps IMU angle or time based - figure it out)\nreturn to auto traversal when done"
      }
      frame "Avoid Right" {
        # "Subroutine for driving counter-clockwise around an obstacle (go right around an obstacle) remain in this routine until completion (perhaps IMU angle or time based - figure it out)\nreturn to auto traversal when done"
      }
      frame "Return to Trench" {
        # "Use drivetrain to return to the trench\nWe know that the distance has been traveled based upon IMU displacement data"
      }
      frame "EXC Deploy" {
        # "watch current on \ndeployment lin acts"
        # "Switch back to manual if button for it pressed"
        # "During testing, \nimmediately go \nback to manual after \ndeployed. For full auto,\nwill be switched to \nEXC excavate"
        # "Use linear actuators and bucket ladder NEOs to deploy the exc bucket ladder\nKnow that deployment is done once linear actuator position corresponding to extension is reached\nOnce deployment is complete, move on to excavating"
        n76 = Greater Or Equal?(x=w456, y=2.05) -> (x >= y?=w487:bool)
        n77 = Greater Or Equal?(x=w464, y=2.01) -> (x >= y?=w486:bool)
        n78 = Greater?(x=w460, y=5.0) -> (0:w454:bool)
        n79 = Index Array(array=w494, index=0) -> (element=w492:bool)
        n80 = In Range and Coerce(upper limit=1.599, x=w456, lower limit=1.5) -> (In Range?=w473:bool)  [unwired: 1 out]
        n81 = Greater?(x=w456, y=1.5) -> (0:w461:bool)
        n82 = And(x=w487, y=w486) -> (x .and. y?=w453:bool)
        n83 = In Range and Coerce(upper limit=1.799, x=w456, lower limit=1.6) -> (In Range?=w477:bool)  [unwired: 1 out]
        n84 = Or(x=w454, y=w453) -> (x .or. y?=w452:bool)
        n85 = Select(t=0.75, s=w473, f=1.0) -> (s? t:f=w470:dbl)
        n86 = Select(t=myStates."Manual Control", s=w452, f=w457) -> (s? t:f=w485:T2)
        n87 = In Range and Coerce(upper limit=2.05, x=w456, lower limit=1.8) -> (In Range?=w481:bool)  [unwired: 1 out]
        n88 = Select(t=0.35, s=w477, f=w470) -> (s? t:f=w476:dbl)
        n89 = Select(t=myStates."Manual Control", s=w492, f=w485) -> (s? t:f=w490:T2)
        n90 = Greater Or Equal?(x=w456, y=2.05) -> (x >= y?=w468:bool)
        n91 = Select(t=0.2, s=w481, f=w476) -> (s? t:f=w466:dbl)
        n92 = Select(t=0.0, s=w468, f=w466) -> (s? t:f=w462:dbl)
        n93 = Select(t=0.65 ("value"), s=w461, f=0.0) -> (s? t:f=w455:dbl)
      }
      frame "EXC Excavate" {
        # "come up with a way to count how long we are excavating and use that to \ngenerate  a function that estimates how much regolith we have excavated"
        # "Run bucket ladder to collect regolith\nremain in this state until one of several volume thresholds have been reached\nthreshold for indexing hopper, reaching this threshold x times indicates full hopper - go to exc retract\nthreshold for inching forward"
      }
      frame "EXC Inch" {
        # "Convert from wheel velocity to\nshaft speedthe sensor sees: \n(Gear ratio * 60) / (2 * pi * wheel radius)"
        # "Velocity we want"
        # "Temporarily using this state to test driving forward slowly autonomously"
        # "use drivetrain to drive forward slowly periodically to position for more regolith\nknow that inching is done based on IMU displacement\nreturn to excavating once distance reached"
        n94 = Unbundle By Name(w526) -> ("Displacement X"=w525:dbl, "Displacement Y"=w524:dbl, "Displacement Z"=w523:dbl)
        n95 = Compound Arithmetic op=ADD(w525, w524, w523) -> (w522:dbl)
        n96 = Greater Or Equal?(x=w522, y=1.0) -> (x >= y?=w531:bool)
        n97 = Multiply(x=-0.05, y=6820.93) -> (x*y=w533:dbl)
        n98 = call-poly <vilib>:"NT Write Value.vi"("value"=w522, "name"="NAVX Dist Y") -> ()  [unwired: 9 in, 1 out]
        n99 = Select(t=myStates."Manual Control", s=w531, f=w529) -> (s? t:f=w528:T2)
      }
      frame "EXC Index" {
        # "Index hopper flat belt periodically to fill hopper volume\nKnow that index is complete based on motor position difference\nonce done go back to excavating"
      }
      frame "EXC Retract" {
        # "Zero navx displacement before leaving state"
        # "Use linear actuators and bucket ladder NEOs to retract the exc bucket ladder\nKnow that retraction is done once linear actuator position corresponding to extension is reached\nOnce retraction is complete, move on to drive to dep or manual"
        n100 = Greater?(x=w587, y=0.28) -> (0:w592:bool)
        n101 = Greater?(x=w589, y=0.3) -> (0:w593:bool)
        n102 = Greater?(x=w589, y=1.6) -> (0:w585:bool)
        n103 = Greater?(x=w587, y=1.56) -> (0:w584:bool)
        n104 = Index Array(array=w576, index=0) -> (element=w569:bool)
        n105 = And(x=w593, y=w592) -> (x .and. y?=w570:bool)
        n106 = Not(x=w570) -> (.not. x?=w571:bool)
        n107 = Select(t=1.0, s=w570, f=0.0) -> (s? t:f=w582:dbl)
        n108 = Or(x=w569, y=w571) -> (x .or. y?=w568:bool)
        n109 = And(x=w585, y=w584) -> (x .and. y?=w580:bool)
        n110 = Select(t=0.5, s=w580, f=w582) -> (s? t:f=w581:dbl)
        n111 = Select(t=myStates."Manual Control", s=w568, f=w573) -> (s? t:f=w572:T2)
        n112 = Select(t=-0.3, s=w580, f=0.0) -> (s? t:f=w577:dbl)
        n113 = call <vilib>:"Zero Displacement.vi"("Zero"=TRUE) -> ()  [unwired: 11 in]
      }
      frame "Drive to Dep" {
        # "Zero navx displacement before leaving state"
        # "Drive to EXC-DEP border (distance from trench to border)\nOnce there, move to Approach berm"
        n114 = call <vilib>:"Zero Displacement.vi"("Zero"=TRUE) -> ()  [unwired: 11 in]
      }
      frame "Approach Berm" {
        # "Zero navx displacement before leaving state"
        # "Drive from EXC-DEP border to berm location.\nUse color sensors the first time to ensure we are lined up with the berm itself\nKnow we are done based on distance traveled and color sensor feedback\nOnce we are there move to HAD deploy"
        n115 = call <vilib>:"Zero Displacement.vi"("Zero"=TRUE) -> ()  [unwired: 11 in]
      }
      frame "HAD Deploy" {
        # "1.68"
        # "1.54"
        # "probably want to deploy during approach - do tasks in parallel"
        # "Ask Nick and Karson where the lin act feedback value comes from - how to read it"
        # "Use linear actuators to deploy HAD bucket ladder.\nCompletion is known once linear actuators reach predetermined position"
        n116 = Greater Or Equal?(x=w659, y=1.54) -> (x >= y?=w655:bool)
        n117 = Greater Or Equal?(x=w656, y=1.68) -> (x >= y?=w654:bool)
        n118 = Index Array(array=w651, index=0) -> (element=w647:bool)
        n119 = And(x=w655, y=w654) -> (x .and. y?=w648:bool)
        n120 = Or(x=w647, y=w648) -> (x .or. y?=w646:bool)
        n121 = Select(t=myStates."Manual Control", s=w646, f=w650) -> (s? t:f=w649:T2)
      }
      frame "HAD Deposit" {
        # "Run flat belt and bucket ladder to deposit regolith into berm.\nKnow that deposition is done via testing averages - takes about XX full \nrotations of the flat belt before all the regolith has been deposited"
      }
      frame "HAD Retract" {
        # "Ask Nick and Karson where the lin act feedback value comes from - how to read it"
        # "Use linear actuators to retract HAD bucket ladder.\nCompletion is known once linear actuators reach predetermined position"
        n122 = Less?(x=w700, y=0.3) -> (x < y?=w698:bool)
        n123 = Less?(x=w703, y=0.3) -> (x < y?=w699:bool)
        n124 = Index Array(array=w706, index=0) -> (element=w704:bool)
        n125 = And(x=w699, y=w698) -> (x .and. y?=w697:bool)
        n126 = Or(x=w704, y=w697) -> (x .or. y?=w696:bool)
        n127 = Select(t=myStates."Manual Control", s=w696, f=w694) -> (s? t:f=w693:T2)
      }
      frame "Return to EXC" {
        # "Drive back to EXC-DEP border using IMU distance data recorded during approach berm"
      }
    }
    n128 = local read "Drivetrain Currents"() -> (w52:dbl[])
    n129 = call-poly <vilib>:"NT Write Value.vi"("value"=w89, "name"="Current State") -> ()  [unwired: 9 in, 1 out]
    n130 = call-poly <vilib>:"NT Read Value.vi"("default value"=FALSE, "name"="Traction Control") -> ("value"=w46:bool)  [unwired: 7 in, 2 out]
    n131 = Index Array(array=w52) -> (element #1=w51:dbl, element #2=w50:dbl, element #3=w49:dbl, element #4=w48:dbl)  [unwired: 4 in]
    n132 = call <vilib>:"WPI_Power Get PD Currents.vi"("PD Channel"=1) -> ("current (A)"=w25:dbl)  [unwired: 11 in, 3 out]
    n133 = call <vilib>:"WPI_Power Get PD Currents.vi"("PD Channel"=2) -> ("current (A)"=w23:dbl)  [unwired: 11 in, 3 out]
    n134 = call <vilib>:"WPI_Power Get PD Currents.vi"("PD Channel"=12) -> ("current (A)"=w20:dbl)  [unwired: 11 in, 3 out]
    n135 = call <vilib>:"WPI_Power Get PD Currents.vi"("PD Channel"=14) -> ("current (A)"=w19:dbl)  [unwired: 11 in, 3 out]
    n136 = case shown="True" w46 {
      tunnel: [w208 w227] -> w40
      tunnel: [w207 w226] -> w39
      tunnel: [w206 w225] -> w45
      tunnel: [w205 w224] -> w44
      tunnel: [w202 w223] -> w43
      tunnel: [w204 w222] -> w42
      tunnel: [w203 w221] -> w38
      tunnel: w59 -> [w208 w220]
      tunnel: w58 -> [w207 w219]
      tunnel: w57 -> [w206 w218]
      tunnel: w56 -> [w205 w217]
      tunnel: w55 -> [w202 w216]
      tunnel: w54 -> [w204 w215]
      tunnel: w53 -> [w203 w214]
      tunnel: w51 -> [_ w213]
      tunnel: w50 -> [_ w212]
      tunnel: w49 -> [_ w211]
      tunnel: w48 -> [_ w210]
      frame False {
      }
      frame True {
        n137 = Bundle(w220, w219, w218, "Left axis value"=w217, "Right axis value"=w216, w215, "Enum"=w214, "current (A)"=w213, "current (A)"=w212, "current (A)"=w211, "current (A)"=w210) -> (w209:T16)  [unwired: 1 in]
        n138 = call "SlipControl.vi"("Input Cluster"=w209) -> ("Output Cluster"=w228:T17)  [unwired: 10 in]
        n139 = Unbundle By Name(w228) -> ("Want to Drive Out"=w227:bool[], "Time Out"=w226:dbl, "Front Left Speed Out"=w225:dbl, "Back Left Speed Out"=w224:dbl, "Front Right Speed Out"=w223:dbl, "Back Right Speed Out"=w222:dbl, "State Out"=w221:T1)
      }
    }
    n140 = Build Array(w25, w23, w20, w19) -> (→"Drivetrain Currents":dbl[])
    n141 = call-poly <vilib>:"NT Write Value.vi"("value"=w25, "name"="FLD Current") -> ()  [unwired: 9 in, 1 out]
    n142 = call-poly <vilib>:"NT Write Value.vi"("value"=w23, "name"="BLD Current") -> ()  [unwired: 9 in, 1 out]
    n143 = call-poly <vilib>:"NT Write Value.vi"("value"=w20, "name"="FRD Current") -> ()  [unwired: 9 in, 1 out]
    n144 = call-poly <vilib>:"NT Write Value.vi"("value"=w19, "name"="BRD Current") -> ()  [unwired: 9 in, 1 out]
    n145 = global read "Robot Global Data.vi" "Robot Mode"() -> (w97:T8)
    n146 = Equal?(x=w97, y=WPI_DriverStationRobotMode2."Teleop Enabled") -> (x = y?=w41:bool)
    n147 = case shown="True" w41 {
      tunnel: [0.0 ("Output") w258] -> w138
      tunnel: w149 -> [_ w258]
      tunnel: [FALSE ("Buttons[0]") w257] -> w137
      tunnel: w148 -> [_ w257]
      tunnel: [0.0 ("f") w251] -> w136
      tunnel: w147 -> [_ w251]
      tunnel: [FALSE ("Buttons[1]") w256] -> w135
      tunnel: w146 -> [_ w256]
      tunnel: [0.0 ("f") w250] -> w134
      tunnel: w145 -> [_ w250]
      tunnel: [0.0 ("f") w255] -> w133
      tunnel: w144 -> [_ w255]
      tunnel: [0.0 ("f") w254] -> w132
      tunnel: w143 -> [_ w254]
      tunnel: [FALSE ("Value") w253] -> w131
      tunnel: w142 -> [_ w253]
      tunnel: [0.0 ("f") w248] -> w130
      tunnel: w141 -> [_ w248]
      tunnel: [FALSE ("Value") w252] -> w129
      tunnel: w140 -> [_ w252]
      tunnel: [0.0 ("f") w249] -> w128
      tunnel: w139 -> [_ w249]
      tunnel: [0.0 ("Setpoint") w247] -> w93
      tunnel: [0.0 ("Setpoint") w246] -> w92
      tunnel: [0.0 ("Setpoint") w245] -> w91
      tunnel: [0.0 ("Setpoint") w244] -> w90
      tunnel: w45 -> [_ w247]
      tunnel: w44 -> [_ w246]
      tunnel: w43 -> [_ w245]
      tunnel: w42 -> [_ w244]
      frame False {
      }
      frame True {
      }
    }
    n148 = call <vilib>:"WPI_MotorControlRefNum Registry Get.vi"("refnum name"="Front Left Drive") -> ("error out"=w80:errorcluster, "MotorControlDevRef"=w79:T18)  [unwired: 9 in]
    n149 = call <vilib>:"WPI_MotorControlRefNum Registry Get.vi"("refnum name"="Back Left Drive") -> ("error out"=w83:errorcluster, "MotorControlDevRef"=w84:T18)  [unwired: 9 in]
    n150 = call <vilib>:"WPI_MotorControlRefNum Registry Get.vi"("refnum name"="Back Right Drive") -> ("error out"=w68:errorcluster, "MotorControlDevRef"=w67:T18)  [unwired: 9 in]
    n151 = call <vilib>:"WPI_MotorControlRefNum Registry Get.vi"("refnum name"="Front Right Drive") -> ("error out"=w71:errorcluster, "MotorControlDevRef"=w72:T18)  [unwired: 9 in]
    n152 = call <vilib>:"WPI_MotorControlRefNum Registry Get.vi"("refnum name"="EXC Bucket Ladder") -> ("error out"=w119:errorcluster, "MotorControlDevRef"=w118:T18)  [unwired: 9 in]
    n153 = call <vilib>:"WPI_DigitalOutputRefNum Registry Get.vi"("refnum name"="EXC Deploy Left DIR") -> ("error out"=w198:errorcluster, "DigitalOutputDevRef"=w197:T23)  [unwired: 9 in]
    n154 = call <vilib>:"WPI_DigitalOutputRefNum Registry Get.vi"("refnum name"="EXC Deploy Left VEL") -> ("error out"=w172:errorcluster, "DigitalOutputDevRef"=w171:T23)  [unwired: 9 in]
    n155 = call <vilib>:"WPI_DigitalOutputRefNum Registry Get.vi"("refnum name"="EXC Deploy Right DIR") -> ("error out"=w191:errorcluster, "DigitalOutputDevRef"=w192:T23)  [unwired: 9 in]
    n156 = Equal?(x=WPI_DriverStationRobotMode2."Teleop Disabled" ("y"), y=w97) -> (x = y?=w107:bool)
    n157 = call <vilib>:"WPI_DigitalOutputRefNum Registry Get.vi"("refnum name"="EXC Deploy Right VEL") -> ("error out"=w190:errorcluster, "DigitalOutputDevRef"=w189:T23)  [unwired: 9 in]
    n158 = call <vilib>:"WPI_MotorControlRefNum Registry Get.vi"("refnum name"="HAD Flat Belt") -> ("error out"=w175:errorcluster, "MotorControlDevRef"=w176:T18)  [unwired: 9 in]
    n159 = call <vilib>:"WPI_MotorControlRefNum Registry Get.vi"("refnum name"="HAD Bucket Ladder") -> ("MotorControlDevRef"=w174:T18)  [unwired: 9 in, 1 out]
    n160 = call <vilib>:"WPI_DigitalOutputRefNum Registry Get.vi"("refnum name"="HAD Deploy Left DIR") -> ("error out"=w177:errorcluster, "DigitalOutputDevRef"=w178:T23)  [unwired: 9 in]
    n161 = call <vilib>:"WPI_DigitalOutputRefNum Registry Get.vi"("refnum name"="HAD Deploy Left VEL") -> ("error out"=w185:errorcluster, "DigitalOutputDevRef"=w186:T23)  [unwired: 9 in]
    n162 = call <vilib>:"WPI_DigitalOutputRefNum Registry Get.vi"("refnum name"="HAD Deploy Right DIR") -> ("error out"=w184:errorcluster, "DigitalOutputDevRef"=w183:T23)  [unwired: 9 in]
    n163 = call <vilib>:"WPI_DigitalOutputRefNum Registry Get.vi"("refnum name"="HAD Deploy Right VEL") -> ("error out"=w187:errorcluster, "DigitalOutputDevRef"=w188:T23)  [unwired: 9 in]
    n164 = call <vilib>:"WPI_MotorControlSetOutput.vi"("error in (no error)"=w119, "Output"=w138, "MotorControlDevRef"=w118) -> ("error out"=w98:errorcluster, "MotorControlDevRef"=w99:T18)  [unwired: 6 in, 1 out]
    n165 = call <vilib>:"WPI_DigitalOutputSetValue.vi"("error in (no error)"=w198, "Value"=w137, "DigitalOutputDevRef"=w197) -> ()  [unwired: 7 in, 2 out]
    n166 = call <vilib>:"WPI_DigitalOutputGeneratePWM.vi"("error in (no error)"=w172, "PWM Duty Cycle"=w136, "DigitalOutputDevRef"=w171) -> ()  [unwired: 7 in, 2 out]
    n167 = call <vilib>:"WPI_DigitalOutputSetValue.vi"("error in (no error)"=w191, "Value"=w135, "DigitalOutputDevRef"=w192) -> ()  [unwired: 7 in, 2 out]
    n168 = call <vilib>:"Spark MAX Set Output Advanced.vi"("error in (no error)"=w80, "Control Mode"=Spark_MAX_Control_Type."Velocity", "Setpoint"=w93, "MotorControlDevRef"=w79) -> ("error out"=w75:errorcluster, "MotorControlDevRef"=w76:T18)  [unwired: 6 in]
    n169 = call <vilib>:"Spark MAX Set Output Advanced.vi"("error in (no error)"=w83, "Control Mode"=Spark_MAX_Control_Type."Velocity", "Setpoint"=w92, "MotorControlDevRef"=w84) -> ("error out"=w81:errorcluster, "MotorControlDevRef"=w82:T18)  [unwired: 6 in]
    n170 = call <vilib>:"WPI_DigitalOutputGeneratePWM.vi"("error in (no error)"=w190, "PWM Duty Cycle"=w134, "DigitalOutputDevRef"=w189) -> ()  [unwired: 7 in, 2 out]
    n171 = call <vilib>:"WPI_MotorControlSetOutput.vi"("error in (no error)"=w175, "Output"=w133, "MotorControlDevRef"=w176) -> ("error out"=w102:errorcluster, "MotorControlDevRef"=w103:T18)  [unwired: 6 in, 1 out]
    n172 = call <vilib>:"Spark MAX Set Output Advanced.vi"("error in (no error)"=w68, "Control Mode"=Spark_MAX_Control_Type."Velocity", "Setpoint"=w90, "MotorControlDevRef"=w67) -> ("error out"=w64:errorcluster, "MotorControlDevRef"=w63:T18)  [unwired: 6 in]
    n173 = call <vilib>:"WPI_MotorControlSetOutput.vi"("Output"=w132, "MotorControlDevRef"=w174) -> ()  [unwired: 7 in, 3 out]
    n174 = call <vilib>:"Spark MAX Set Output Advanced.vi"("error in (no error)"=w71, "Control Mode"=Spark_MAX_Control_Type."Velocity", "Setpoint"=w91, "MotorControlDevRef"=w72) -> ("error out"=w69:errorcluster, "MotorControlDevRef"=w70:T18)  [unwired: 6 in]
    n175 = call <vilib>:"WPI_DigitalOutputSetValue.vi"("error in (no error)"=w177, "Value"=w131, "DigitalOutputDevRef"=w178) -> ()  [unwired: 7 in, 2 out]
    n176 = call <vilib>:"WPI_DigitalOutputSetValue.vi"("error in (no error)"=w184, "Value"=w129, "DigitalOutputDevRef"=w183) -> ()  [unwired: 7 in, 2 out]
    n177 = call <vilib>:"WPI_DigitalOutputGeneratePWM.vi"("error in (no error)"=w185, "PWM Duty Cycle"=w130, "DigitalOutputDevRef"=w186) -> ()  [unwired: 7 in, 2 out]
    n178 = call <vilib>:"WPI_DigitalOutputGeneratePWM.vi"("error in (no error)"=w187, "PWM Duty Cycle"=w128, "DigitalOutputDevRef"=w188) -> ()  [unwired: 7 in, 2 out]
    n179 = Select(t=myStates."Manual Control", s=w107, f=w106) -> (s? t:f=w105:T2)
    n180 = call <vilib>:"Spark MAX Get Sensor Position.vi"("error in (no error)"=w98, "MotorControlDevRef in"=w99) -> ("Sensor Position"=w95:dbl)  [unwired: 6 in, 3 out]
    n181 = call <vilib>:"Spark MAX Get Sensor Position.vi"("error in (no error)"=w102, "MotorControlDevRef in"=w103) -> ("Sensor Position"=w101:dbl)  [unwired: 6 in, 3 out]
    n182 = call <vilib>:"Spark MAX Get Sensor Velocity.vi"("error in (no error)"=w64, "MotorControlDevRef in"=w63) -> ()  [unwired: 6 in, 4 out]
    n183 = call <vilib>:"Spark MAX Get Sensor Velocity.vi"("error in (no error)"=w69, "MotorControlDevRef in"=w70) -> ()  [unwired: 6 in, 4 out]
    n184 = call <vilib>:"Spark MAX Get Sensor Velocity.vi"("error in (no error)"=w81, "MotorControlDevRef in"=w82) -> ()  [unwired: 6 in, 4 out]
    n185 = call <vilib>:"Spark MAX Get Sensor Velocity.vi"("error in (no error)"=w75, "MotorControlDevRef in"=w76) -> ()  [unwired: 6 in, 4 out]
    n186 = Divide(x=w95, y=-193.0) -> (x/y=w94:dbl)
    n187 = call-poly <vilib>:"NT Write Value.vi"("value"=w101, "name"="Flat Belt Position") -> ()  [unwired: 9 in, 1 out]
    n188 = call-poly <vilib>:"NT Write Value.vi"("value"=w94, "name"="EXC BL Position") -> ()  [unwired: 9 in, 1 out]
    n189 = Wait (ms)(milliseconds to wait=u32 100) -> ()  [unwired: 1 out]
  }
  n190 = while {
    shift-right: [w759] -> _
    shift-left: _ -> [w785]
    shift-right: [w758] -> _
    shift-left: _ -> [w781]
    shift-left: _ -> [w780]
    shift-left: _ -> [w779]
    shift-left: _ -> [w778]
    shift-left: _ -> [w784]
    shift-left: _ -> [w783]
    shift-left: _ -> [w782]
    tunnel: w8 -> [w771]
    tunnel: w7 -> [w770]
    shift-left: _ -> [w769]
    shift-left: _ -> [w768]
    shift-left: _ -> [w767]
    shift-left: _ -> [w766]
    shift-left: _ -> [w765]
    shift-left: _ -> [w764]
    shift-left: _ -> [w763]
    shift-left: _ -> [w762]
    shift-left: _ -> [w761]
    shift-left: _ -> [w760]
    tunnel: w6 -> [w756]
    tunnel: w5 -> [w755]
    shift-right: [w754] -> _
    shift-left: _ -> [w753]
    shift-left: _ -> [w752]
    shift-left: _ -> [w751]
    shift-left: _ -> [w750]
    shift-left: _ -> [w749]
    shift-right: [w746] -> _
    shift-left: _ -> [w745]
    shift-left: _ -> [w744]
    shift-left: _ -> [w743]
    shift-left: _ -> [w742]
    shift-left: _ -> [w741]
    stop <- FALSE stop-if-true
    # "creating/writing a variable"
    # "Running Average of linear actuator\nvoltage readings. The purpose is to\navoid issues with reading fluctuation"
    n191 = call <vilib>:"WPI_AnalogChannelGetVoltage.vi"("AIDeviceRef"=w771) -> ("Voltage"=w759:dbl)  [unwired: 8 in, 2 out]
    n192 = call <vilib>:"WPI_AnalogChannelGetVoltage.vi"("AIDeviceRef"=w756) -> ("Voltage"=w754:dbl)  [unwired: 8 in, 2 out]
    n193 = call <vilib>:"WPI_AnalogChannelGetVoltage.vi"("AIDeviceRef"=w770) -> ("Voltage"=w758:dbl)  [unwired: 8 in, 2 out]
    n194 = call <vilib>:"WPI_AnalogChannelGetVoltage.vi"("AIDeviceRef"=w755) -> ("Voltage"=w746:dbl)  [unwired: 8 in, 2 out]
    n195 = Compound Arithmetic op=ADD(w746, w745, w744, w743, w742, w741) -> (w739:dbl)
    n196 = Compound Arithmetic op=ADD(w754, w753, w752, w751, w750, w749) -> (w748:dbl)
    n197 = Compound Arithmetic op=ADD(w759, w785, w784, w783, w782, w766, w765, w764, w761, w760) -> (w777:dbl)
    n198 = Compound Arithmetic op=ADD(w758, w781, w780, w779, w778, w769, w768, w767, w763, w762) -> (w773:dbl)
    n199 = Divide(x=w748, y=6.0) -> (x/y=→"DEP Left Running Ave":dbl)
    n200 = Divide(x=w739, y=6.0) -> (x/y=→"DEP Right Running Ave":dbl)
    n201 = Divide(x=w777, y=10.0) -> (x/y=→"EXC Left Running Ave":dbl)
    n202 = Divide(x=w773, y=10.0) -> (x/y=→"EXC Right Running Ave":dbl)
    n203 = Wait (ms)(milliseconds to wait=u32 75) -> ()  [unwired: 1 out]
  }
  n204 = disable-structure shown="Disabled" {
    disable-tunnel: _ -> [w788 _]
    disable-tunnel: _ -> [w787 _]
    frame Disabled {
      n205 = call <vilib>:"WPI_RobotDriveRefNum Registry Get.vi"("refnum name"="Left and Right Motors") -> ("error out"=w793:errorcluster, "RobotDriveDevRef"=w792:T24)  [unwired: 9 in]
      n206 = call <vilib>:"WPI_RobotDriveTankDrive.vi"("error in (no error)"=w793, "Right axis value"=w787, "Left axis value"=w788, "RobotDriveDevRef"=w792) -> ("Motor Values"=w789:dbl[])  [unwired: 5 in, 2 out]
      n207 = call-poly <vilib>:"NT Write Value.vi"("value"=w789, "name"="RobotDrive Motors" ("Name")) -> ()  [unwired: 9 in, 1 out]
    }
    frame Enabled {
    }
  }
